vi "Generate Report.vi"(11 "Data In":T1={"Impulse Positions"=[], "No. Imp"=0, "Parameter Time Series"=[], "Parameter Impuls Series"=[], "Experiment Parameters"={"Freq"=0.0, "Vel"=0, "Acc"=0, "Stimulus"=""}, "Autosort File"=refnum, "Data File"={"Data Channels"=[], "Sample Rate"=0, "Channel List"=[]}, "Experiment data path"=path "/Macintosh HD/Users/patrick/Studium/Diploma Thesis/Data Analysis", "Image data path"=path "/Macintosh HD/Users/patrick/Studium/Diploma Thesis/Data Analysis", "LVS data path"=path "/Macintosh HD/Users/patrick/Studium/Diploma Thesis/Data Analysis", "Raw copy path"=path "/Macintosh HD/Users/patrick/Studium/Diploma Thesis/Data Analysis", "filename"="No file selected", "desaccading parameters"={"Tolerance"=0, "Acc Range"=0.0, "Sample Rate"=0, "Impulse Plane 2"=enum."Other", "Impulse dir"=FALSE}, "Experiment Parameters 2"={"Subject"="", "Strain"="", "Rotation plane"="", "Experimenter"="", "Trial"=0.0, "Time"=0.0}, "Excel"={"Excel._Application"=refnum, "Use Excel"=FALSE, "Worksheet SINE"=refnum, "Row SINE"=0, "Worksheet TRANS"=refnum, "Row TRANS"=0}, "Session Config File"=refnum, "Autosort Parameter Set"=1, "EMA Version"="", "desacc "={"Threshold 1 [Acc]"=7000.0, "Threshold 2 [% of TH1]"=60, "tolerance"=3, "Search WD "=0.1, " always use TH2"=FALSE, "Range"=2.0, "Max time"=120.0, "Min time"=20.0, "Velocity Threshold"=150}, "Cycle Nr for Saccades"={"POS"=0, "NEG"=0}, "calibration name"="No file selected", "Excel"=refnum} {"Parameter Time Series"."time offset" format="%.3f"; "Parameter Time Series"."Gain" format="%.1f"; "Parameter Time Series"."Offset" format="%.1f"; "Parameter Time Series"."List 1" items=["Motor-Pos", "Motor-Vel", "Lx Position-in-Head", "Ly Position-in-Head", "Lz Position-in-Head", "Lx Velocity-in-Head", "Ly Velocity-in-Head", "Lz Velocity-in-Head", "Ll Velocity-in-Head", "Lr Velocity-in-Head", "Lx Accel-in-Head", "Ly Accel-in-Head", "Lz Accel-in-Head", "Rx Position-in-Head", "Ry Position-in-Head", "Rz Position-in-Head", "Rx Velocity-in-Head", "Ry Velocity-in-Head", "Rz Velocity-in-Head", "Rl Velocity-in-Head", "Rr Velocity-in-Head", "Rx Accel-in-Head", "Ry Accel-in-Head", "Rz Accel-in-Head", "Global Trigger", "", "", ""]; "Parameter Impuls Series"."Gain" format="%.1f"; "Parameter Impuls Series"."Offset" format="%.1f"}) -> (3 "Data Out":T1={"Impulse Positions"=[], "No. Imp"=0, "Parameter Time Series"=[], "Parameter Impuls Series"=[], "Experiment Parameters"={"Freq"=0.0, "Vel"=0, "Acc"=0, "Stimulus"=""}, "Autosort File"=refnum, "Data File"={"Data Channels"=[], "Sample Rate"=0, "Channel List"=[]}, "Experiment data path"=path "/Macintosh HD/Users/patrick/Studium/Diploma Thesis/Data Analysis", "Image data path"=path "/Macintosh HD/Users/patrick/Studium/Diploma Thesis/Data Analysis", "LVS data path"=path "/Macintosh HD/Users/patrick/Studium/Diploma Thesis/Data Analysis", "Raw copy path"=path "/Macintosh HD/Users/patrick/Studium/Diploma Thesis/Data Analysis", "filename"="No file selected", "desaccading parameters"={"Tolerance"=0, "Acc Range"=0.0, "Sample Rate"=0, "Impulse Plane 2"=enum."Other", "Impulse dir"=FALSE}, "Experiment Parameters 2"={"Subject"="", "Strain"="", "Rotation plane"="", "Experimenter"="", "Trial"=0.0, "Time"=0.0}, "Excel"={"Excel._Application"=refnum, "Use Excel"=FALSE, "Worksheet SINE"=refnum, "Row SINE"=0, "Worksheet TRANS"=refnum, "Row TRANS"=0}, "Session Config File"=refnum, "Autosort Parameter Set"=1, "EMA Version"="", "desacc "={"Threshold 1 [Acc]"=7000.0, "Threshold 2 [% of TH1]"=60, "tolerance"=3, "Search WD "=0.1, " always use TH2"=FALSE, "Range"=2.0, "Max time"=120.0, "Min time"=20.0, "Velocity Threshold"=150}, "Cycle Nr for Saccades"={"POS"=0, "NEG"=0}, "calibration name"="No file selected", "Excel"=refnum} {"Parameter Time Series"."time offset" format="%.3f"; "Parameter Time Series"."Gain" format="%.1f"; "Parameter Time Series"."Offset" format="%.1f"; "Parameter Time Series"."List 1" items=["Motor-Pos", "Motor-Vel", "Lx Position-in-Head", "Ly Position-in-Head", "Lz Position-in-Head", "Lx Velocity-in-Head", "Ly Velocity-in-Head", "Lz Velocity-in-Head", "Ll Velocity-in-Head", "Lr Velocity-in-Head", "Lx Accel-in-Head", "Ly Accel-in-Head", "Lz Accel-in-Head", "Rx Position-in-Head", "Ry Position-in-Head", "Rz Position-in-Head", "Rx Velocity-in-Head", "Ry Velocity-in-Head", "Rz Velocity-in-Head", "Rl Velocity-in-Head", "Rr Velocity-in-Head", "Rx Accel-in-Head", "Ry Accel-in-Head", "Rz Accel-in-Head", "Global Trigger", "", "", ""]; "Parameter Impuls Series"."Gain" format="%.1f"; "Parameter Impuls Series"."Offset" format="%.1f"})   [LabVIEW 2016, in "generate report.lvlib"]
uses:
  generate report.lvlib
  core/type-defs/TD_Statemachine-Data.ctl
  <userlib>/Import Export/Excel/Excel.lvclass
  core/type-defs/TD_Time Series.ctl
  core/type-defs/TD_Impulse Parameter.ctl
  Enum_Statistical Methods Within Impulses.ctl
  Enum_Statistical Methods Across Impulses.ctl
  Enum_Report State.ctl
  <vilib>/Utility/miscctls.llb/LVRectTypeDef.ctl
  <vilib>/Utility/NIReport.llb/Append Image to Report (path wrap).vi
  <vilib>/Utility/NIReport.llb/Append Report Text (str wrap).vi
  <vilib>/Utility/NIReport.llb/NI_report.lvclass
  comm/impulse/impulse functions.lvlib
  <vilib>/Utility/NIReport.llb/NI_ReportGenerationCore.lvlib
  core/core.lvlib
panel:
  in  "5 PeakVel SD":dbl format="%#_13g"
  in  "5 PeakVel":dbl format="%#_13g"
  in  "4 PeakVel SD":dbl format="%#_13g"
  in  "4 PeakVel":dbl format="%#_13g"
  in  "2 PeakVel":dbl format="%#_13g"
  in  "2 PeakVel SD":dbl format="%#_13g"
  in  "3 PeakVel":dbl format="%#_13g"
  in  "3 PeakVel SD":dbl format="%#_13g"
  in  "1 PeakVel":dbl format="%#_13g"
  in  "1 PeakVel SD":dbl format="%#_13g"
  in  "0 PeakVel SD":dbl format="%#_13g"
  in  "0 PeakVel":dbl format="%#_13g"
  out "5 N":i32
  out "4 N":i32
  out "3 N":i32
  out "2 N":i32
  out "1 N":i32
  out "0 N":i32
  out "Stimulus":string
  out "3 SD":dbl=-0.0 format="%.2f"
  out "2 SD":dbl=-0.0 format="%.2f"
  out "0 SD":dbl=-0.0 format="%.2f"
  out "1 SD":dbl=-0.0 format="%.2f"
  out "4 SD":dbl=-0.0 format="%.2f"
  out "5 SD":dbl=-0.0 format="%.2f"
  out "3 Gain":dbl=nan format="%.2f"
  out "2 Gain":dbl=nan format="%.2f"
  out "0 Gain":dbl=nan format="%.2f"
  out "1 Gain":dbl=nan format="%.2f"
  in  "Patient ID":string
  out "4 Gain":dbl=nan format="%.2f"
  out "5 Gain":dbl=nan format="%.2f"
  out "5":cluster{dbl, dbl, "Impulses":dbl[][]}(graph)={0.0, 2.5, "Impulses"=[]}
  out "3":cluster{dbl, dbl, "Impulses":dbl[][]}(graph)={0.0, 2.5, "Impulses"=[]}
  out "4":cluster{dbl, dbl, "Impulses":dbl[][]}(graph)={0.0, 2.5, "Impulses"=[]}
  out "2":cluster{dbl, dbl, "Impulses":dbl[][]}(graph)={0.0, 2.5, "Impulses"=[]}
  out "1":cluster{dbl, dbl, "Impulses":dbl[][]}(graph)={0.0, 2.5, "Impulses"=[]}
  out "0":cluster{dbl, dbl, "Impulses":dbl[][]}(graph)={0.0, 2.5, "Impulses"=[]}
  in  "Save to Excel (legacy)":bool
  in  "PS - RollPitch":bool
  in  "PS - EyHy":bool
  in  "PS - EyHlr":bool
  in  "PS - All3D":bool
  out "Analysis Required?":bool
  in  "Impulse Group Gain Method":T4
  in  "Impulse Gain Method":T5=enum."Median"
  in  "Save to Excel":bool
  in  "Printer Select":string(combo) caption="Selected Printer"
  in  "print horizontal":bool
  in  "Save to File":bool
  in  "print all":bool
  in  "Graph Properties":T6(array[cluster])=[{"Plot Traces"=[{"Color Box"=6618880, "Boolean"=TRUE, "List 2"=1, "Boolean 2"=FALSE, "Boolean 3"=FALSE, "Offset"=0.0, "Gain"=1.0}, {"Color Box"=4467455, "Boolean"=TRUE, "List 2"=13, "Boolean 2"=TRUE, "Boolean 3"=FALSE, "Offset"=0.0, "Gain"=1.0}, {"Color Box"=16711680, "Boolean"=TRUE, "List 2"=21, "Boolean 2"=TRUE, "Boolean 3"=FALSE, "Offset"=0.0, "Gain"=1.0}], "Gain Calculations"={"Threshold Trace"=1, "Min Thresh/%"=0.2, "Max Thresh/%"=0.8, "Gain calculated by dividing"=13, "Gain Range"=enum."Best Est", "Pre-peak-ms"=30.0, "by"=1}, "Impulse Plane"=enum."Yaw", "Impulse Direction"=TRUE}, {"Plot Traces"=[{"Color Box"=6618880, "Boolean"=TRUE, "List 2"=1, "Boolean 2"=TRUE, "Boolean 3"=FALSE, "Offset"=0.0, "Gain"=1.0}, {"Color Box"=1966335, "Boolean"=TRUE, "List 2"=13, "Boolean 2"=FALSE, "Boolean 3"=FALSE, "Offset"=0.0, "Gain"=1.0}, {"Color Box"=16711680, "Boolean"=TRUE, "List 2"=21, "Boolean 2"=FALSE, "Boolean 3"=FALSE, "Offset"=0.0, "Gain"=1.0}], "Gain Calculations"={"Threshold Trace"=1, "Min Thresh/%"=0.2, "Max Thresh/%"=0.8, "Gain calculated by dividing"=13, "Gain Range"=enum."Best Est", "Pre-peak-ms"=30.0, "by"=1}, "Impulse Plane"=enum."Yaw", "Impulse Direction"=FALSE}, {"Plot Traces"=[{"Color Box"=4652800, "Boolean"=TRUE, "List 2"=6, "Boolean 2"=TRUE, "Boolean 3"=FALSE, "Offset"=0.0, "Gain"=1.0}, {"Color Box"=1966335, "Boolean"=TRUE, "List 2"=14, "Boolean 2"=FALSE, "Boolean 3"=FALSE, "Offset"=0.0, "Gain"=1.0}, {"Color Box"=16722474, "Boolean"=TRUE, "List 2"=22, "Boolean 2"=FALSE, "Boolean 3"=FALSE, "Offset"=0.0, "Gain"=1.0}], "Gain Calculations"={"Threshold Trace"=6, "Min Thresh/%"=0.2, "Max Thresh/%"=0.8, "Gain calculated by dividing"=14, "Gain Range"=enum."Best Est", "Pre-peak-ms"=30.0, "by"=6}, "Impulse Plane"=enum."LARP", "Impulse Direction"=FALSE}, {"Plot Traces"=[{"Color Box"=4652800, "Boolean"=TRUE, "List 2"=7, "Boolean 2"=FALSE, "Boolean 3"=FALSE, "Offset"=0.0, "Gain"=1.0}, {"Color Box"=1966335, "Boolean"=TRUE, "List 2"=15, "Boolean 2"=TRUE, "Boolean 3"=FALSE, "Offset"=0.0, "Gain"=1.0}, {"Color Box"=16722474, "Boolean"=TRUE, "List 2"=23, "Boolean 2"=TRUE, "Boolean 3"=FALSE, "Offset"=0.0, "Gain"=1.0}], "Gain Calculations"={"Threshold Trace"=7, "Min Thresh/%"=0.2, "Max Thresh/%"=0.8, "Gain calculated by dividing"=15, "Gain Range"=enum."Best Est", "Pre-peak-ms"=30.0, "by"=7}, "Impulse Plane"=enum."RALP", "Impulse Direction"=TRUE}, {"Plot Traces"=[{"Color Box"=4652800, "Boolean"=TRUE, "List 2"=7, "Boolean 2"=TRUE, "Boolean 3"=FALSE, "Offset"=0.0, "Gain"=1.0}, {"Color Box"=1966335, "Boolean"=TRUE, "List 2"=15, "Boolean 2"=FALSE, "Boolean 3"=FALSE, "Offset"=0.0, "Gain"=1.0}, {"Color Box"=16722474, "Boolean"=TRUE, "List 2"=23, "Boolean 2"=FALSE, "Boolean 3"=FALSE, "Offset"=0.0, "Gain"=1.0}], "Gain Calculations"={"Threshold Trace"=7, "Min Thresh/%"=0.2, "Max Thresh/%"=0.8, "Gain calculated by dividing"=15, "Gain Range"=enum."Best Est", "Pre-peak-ms"=30.0, "by"=7}, "Impulse Plane"=enum."RALP", "Impulse Direction"=FALSE}, {"Plot Traces"=[{"Color Box"=4652800, "Boolean"=TRUE, "List 2"=6, "Boolean 2"=FALSE, "Boolean 3"=FALSE, "Offset"=0.0, "Gain"=1.0}, {"Color Box"=1966335, "Boolean"=TRUE, "List 2"=14, "Boolean 2"=TRUE, "Boolean 3"=FALSE, "Offset"=0.0, "Gain"=1.0}, {"Color Box"=16722474, "Boolean"=TRUE, "List 2"=22, "Boolean 2"=TRUE, "Boolean 3"=FALSE, "Offset"=0.0, "Gain"=1.0}], "Gain Calculations"={"Threshold Trace"=6, "Min Thresh/%"=0.2, "Max Thresh/%"=0.8, "Gain calculated by dividing"=14, "Gain Range"=enum."Best Est", "Pre-peak-ms"=30.0, "by"=6}, "Impulse Plane"=enum."LARP", "Impulse Direction"=TRUE}] {"Gain Calculations"."by" items=["-", "Hz Velocity-in-Head", "-", "Hy Velocity-in-Head", "-", "Hx Velocity-in-Head", "Hl Velocity-in-Head", "Hr Velocity-in-Head", "-", "Ly Position-in-Head", "Lz Position-in-Head", "-", "Ly Velocity-in-Head", "Lz Velocity-in-Head", "-", "Hx Acceleration-in-Head", "Hy Acceleration-in-Head", "Hz Acceleration-in-Head", "Hl Acceleration-in-Head", "Hr Acceleration-in-Head", "-", "Ly Acceleration-in-Head", "Lz Acceleration-in-Head", "-"]; "Gain Calculations"."Pre-peak-ms" format="%.2f"; "Gain Calculations"."Gain calculated by dividing" items=["-", "Hz Velocity-in-Head", "-", "Hy Velocity-in-Head", "-", "Hx Velocity-in-Head", "Hl Velocity-in-Head", "Hr Velocity-in-Head", "-", "Ly Position-in-Head", "Lz Position-in-Head", "-", "Ly Velocity-in-Head", "Lz Velocity-in-Head", "-", "Hx Acceleration-in-Head", "Hy Acceleration-in-Head", "Hz Acceleration-in-Head", "Hl Acceleration-in-Head", "Hr Acceleration-in-Head", "-", "Ly Acceleration-in-Head", "Lz Acceleration-in-Head", "-"]; "Gain Calculations"."Max Thresh/%" format="%.2f"; "Gain Calculations"."Min Thresh/%" format="%.2f"; "Gain Calculations"."Threshold Trace" items=["-", "Hz Velocity-in-Head", "-", "Hy Velocity-in-Head", "-", "Hx Velocity-in-Head", "Hl Velocity-in-Head", "Hr Velocity-in-Head", "-", "Ly Position-in-Head", "Lz Position-in-Head", "-", "Ly Velocity-in-Head", "Lz Velocity-in-Head", "-", "Hx Acceleration-in-Head", "Hy Acceleration-in-Head", "Hz Acceleration-in-Head", "Hl Acceleration-in-Head", "Hr Acceleration-in-Head", "-", "Ly Acceleration-in-Head", "Lz Acceleration-in-Head", "-"]; "Plot Traces"."Gain" format="%.1f"; "Plot Traces"."Offset" format="%.1f"; "Plot Traces"."List 2" items=["-", "Hz Velocity-in-Head", "-", "Hy Velocity-in-Head", "-", "Hx Velocity-in-Head", "Hl Velocity-in-Head", "Hr Velocity-in-Head", "-", "Ly Position-in-Head", "Lz Position-in-Head", "-", "Ly Velocity-in-Head", "Lz Velocity-in-Head", "-", "Hx Acceleration-in-Head", "Hy Acceleration-in-Head", "Hz Acceleration-in-Head", "Hl Acceleration-in-Head", "Hr Acceleration-in-Head", "-", "Ly Acceleration-in-Head", "Lz Acceleration-in-Head", "-"]}
  # "Canal Plane Responses"
  # "RIGHT"
  # "LEFT"
  # "Horizontal"
  # "Horizontal"
  # "Anterior"
  # "Anterior"
  # "Posterior"
  # "Posterior"
  # "Gain Calculation Presets"
  # "Copyright Americo A. Migliaccio (c) 2002 All Rights Reserved by Author"
  # "Gain Methods for 'Best Est' Calculation"
  # "-"
  # "+"
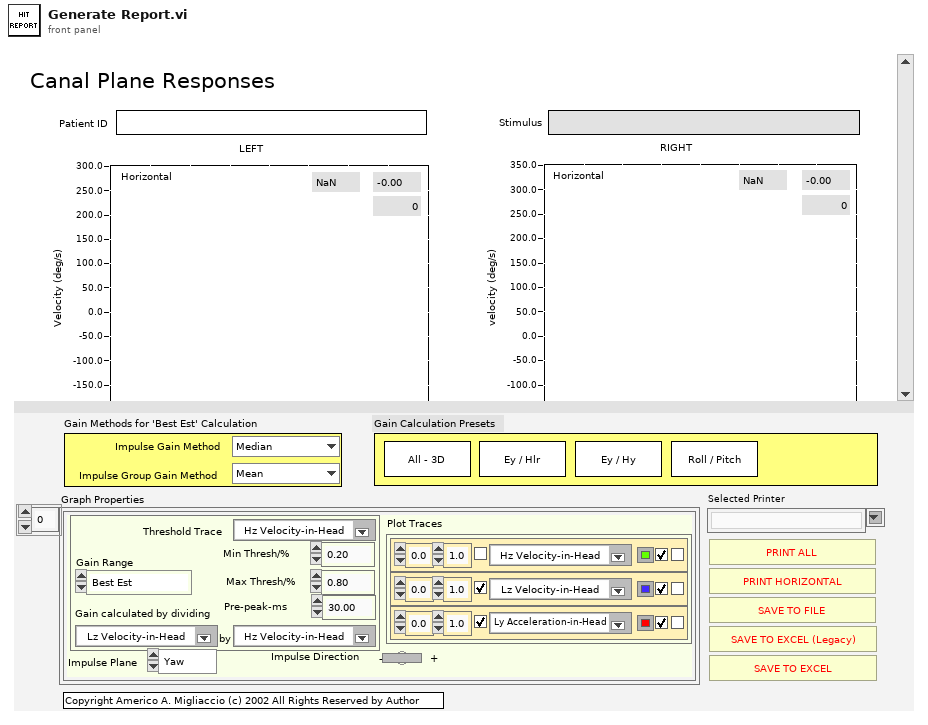
[diagram p1: front panel]
types:
  T1 = typedef "core.lvlib/TD_Statemachine-Data.ctl" = cluster{"Impulse Positions":cluster{"Start":i32, "End":i32, "Impulse Plane":enum16{"Other", "Yaw", "Pitch", "Roll", "LARP", "RALP"}, "Impulse Direction +ve?":bool, "Time offset":i32, "Amplitude offset":dbl}[], "No. Imp":i32, "Parameter Time Series":T2, "Parameter Impuls Series":T3, "Experiment Parameters":cluster{"Freq":dbl, "Vel":i32, "Acc":i32, "Stimulus":string}, "Autosort File":refnum<file>, "Data File":cluster{"Data Channels":dbl[][], "Sample Rate":i32, "Channel List":string[]}, "Experiment data path":path, "Image data path":path, "LVS data path":path, "Raw copy path":path, "filename":string, "desaccading parameters":cluster{"Tolerance":i32, "Acc Range":dbl, "Sample Rate":i32, "Impulse Plane 2":enum16{"Other", "Yaw", "Pitch", "Roll", "LARP", "RALP"}, "Impulse dir":bool}, "Experiment Parameters 2":cluster{"Subject":string, "Strain":string, "Rotation plane":string, "Experimenter":string, "Trial":dbl, "Time":dbl}, "Excel":cluster{"Excel._Application":refnum<k7>, "Use Excel":bool, "Worksheet SINE":refnum<k7>, "Row SINE":i32, "Worksheet TRANS":refnum<k7>, "Row TRANS":i32}, "Session Config File":refnum<file>, "Autosort Parameter Set":i32, "EMA Version":string, "desacc ":cluster{"Threshold 1 [Acc]":dbl, "Threshold 2 [% of TH1]":i32, "tolerance":i32, "Search WD ":dbl, " always use TH2":bool, "Range":dbl, "Max time":dbl, "Min time":dbl, "Velocity Threshold":i32}, "Cycle Nr for Saccades":cluster{"POS":i32, "NEG":i32}, "calibration name":string, "Excel":refnum<class "Excel.lvclass">}
  T2 = typedef "core.lvlib/TD_Time Series.ctl" = cluster{"time offset":dbl, "Offset":dbl, "Gain":dbl, "inverse":bool, "filter data":bool, "dots":bool, "interpolate":bool, "List 1":u16, "Color Box":u32, "Boolean":bool}[]
  T3 = typedef "core.lvlib/TD_Impulse Parameter.ctl" = cluster{"Color":u32, "Visible":bool, "Channel":u16, "Invert":bool, "Desaccade":bool, "Offset":dbl, "Gain":dbl}[]
  T4 = typedef "generate report.lvlib/Enum_Statistical Methods Across Impulses.ctl" = enum16{"Mean", "Median"}
  T5 = typedef "generate report.lvlib/Enum_Statistical Methods Within Impulses.ctl" = enum16{"Max", "Mean", "Median"}
  T6 = cluster{"Plot Traces":cluster{"Color Box":u32, "Boolean":bool, "List 2":u16, "Boolean 2":bool, "Boolean 3":bool, "Offset":dbl, "Gain":dbl}[], "Gain Calculations":cluster{"Threshold Trace":u16, "Min Thresh/%":dbl, "Max Thresh/%":dbl, "Gain calculated by dividing":u16, "Gain Range":enum16{"Peak %", "Best Est", "Thresh"}, "Pre-peak-ms":dbl, "by":u16}, "Impulse Plane":enum16{"Other", "Yaw", "Pitch", "Roll", "LARP", "RALP"}, "Impulse Direction":bool}[]
  T7 = typedef "generate report.lvlib/Enum_Report State.ctl" = enum16{"Idle", "Initialize", "Quit", "Analyze", "Print All", "Print Horizontal", "Save Text File", "Save To Excel", "Save To Excel (legacy)"}
  T8 = enum16{"Standard Report", "HTML", "Word", "Excel"}
  T9 = cluster{"left":i16, "top":i16, "right":i16, "bottom":i16}
  T10 = typedef "LVRectTypeDef.ctl" = cluster{"Left":i16, "Top":i16, "Right":i16, "Bottom":i16}
  T11 = enum16{"open", "replace", "create", "open or create", "replace or create", "replace or create with confirmation"}
  T12 = cluster{"Threshold 1 [Acc]":dbl, "Threshold 2 [% of TH1]":i32, "tolerance":i32, "Search WD ":dbl, " always use TH2":bool, "Range":dbl, "Max time":dbl, "Min time":dbl, "Velocity Threshold":i32}
  T13 = cluster{"Data Channels":dbl[][], "Sample Rate":i32, "Channel List":string[]}
  T14 = cluster{"Start":i32, "End":i32, "Impulse Plane":enum16{"Other", "Yaw", "Pitch", "Roll", "LARP", "RALP"}, "Impulse Direction +ve?":bool, "Time offset":i32, "Amplitude offset":dbl}[]
  T15 = cluster{"Impulse Gain Method":T5, "Impulse Group Gain Method":T4}
  T16 = enum16{"Other", "Yaw", "Pitch", "Roll", "LARP", "RALP"}
  T17 = cluster{"Color Box":u32, "Boolean":bool, "List 2":u16, "Boolean 2":bool, "Boolean 3":bool, "Offset":dbl, "Gain":dbl}[]
  T18 = typedef "imagedata.ctl" = cluster{"image type":i32, "image depth":i32, "image":u8[], "mask":u8[], "colors":u32[], "Rectangle":cluster{"left":i16, "top":i16, "right":i16, "bottom":i16}}
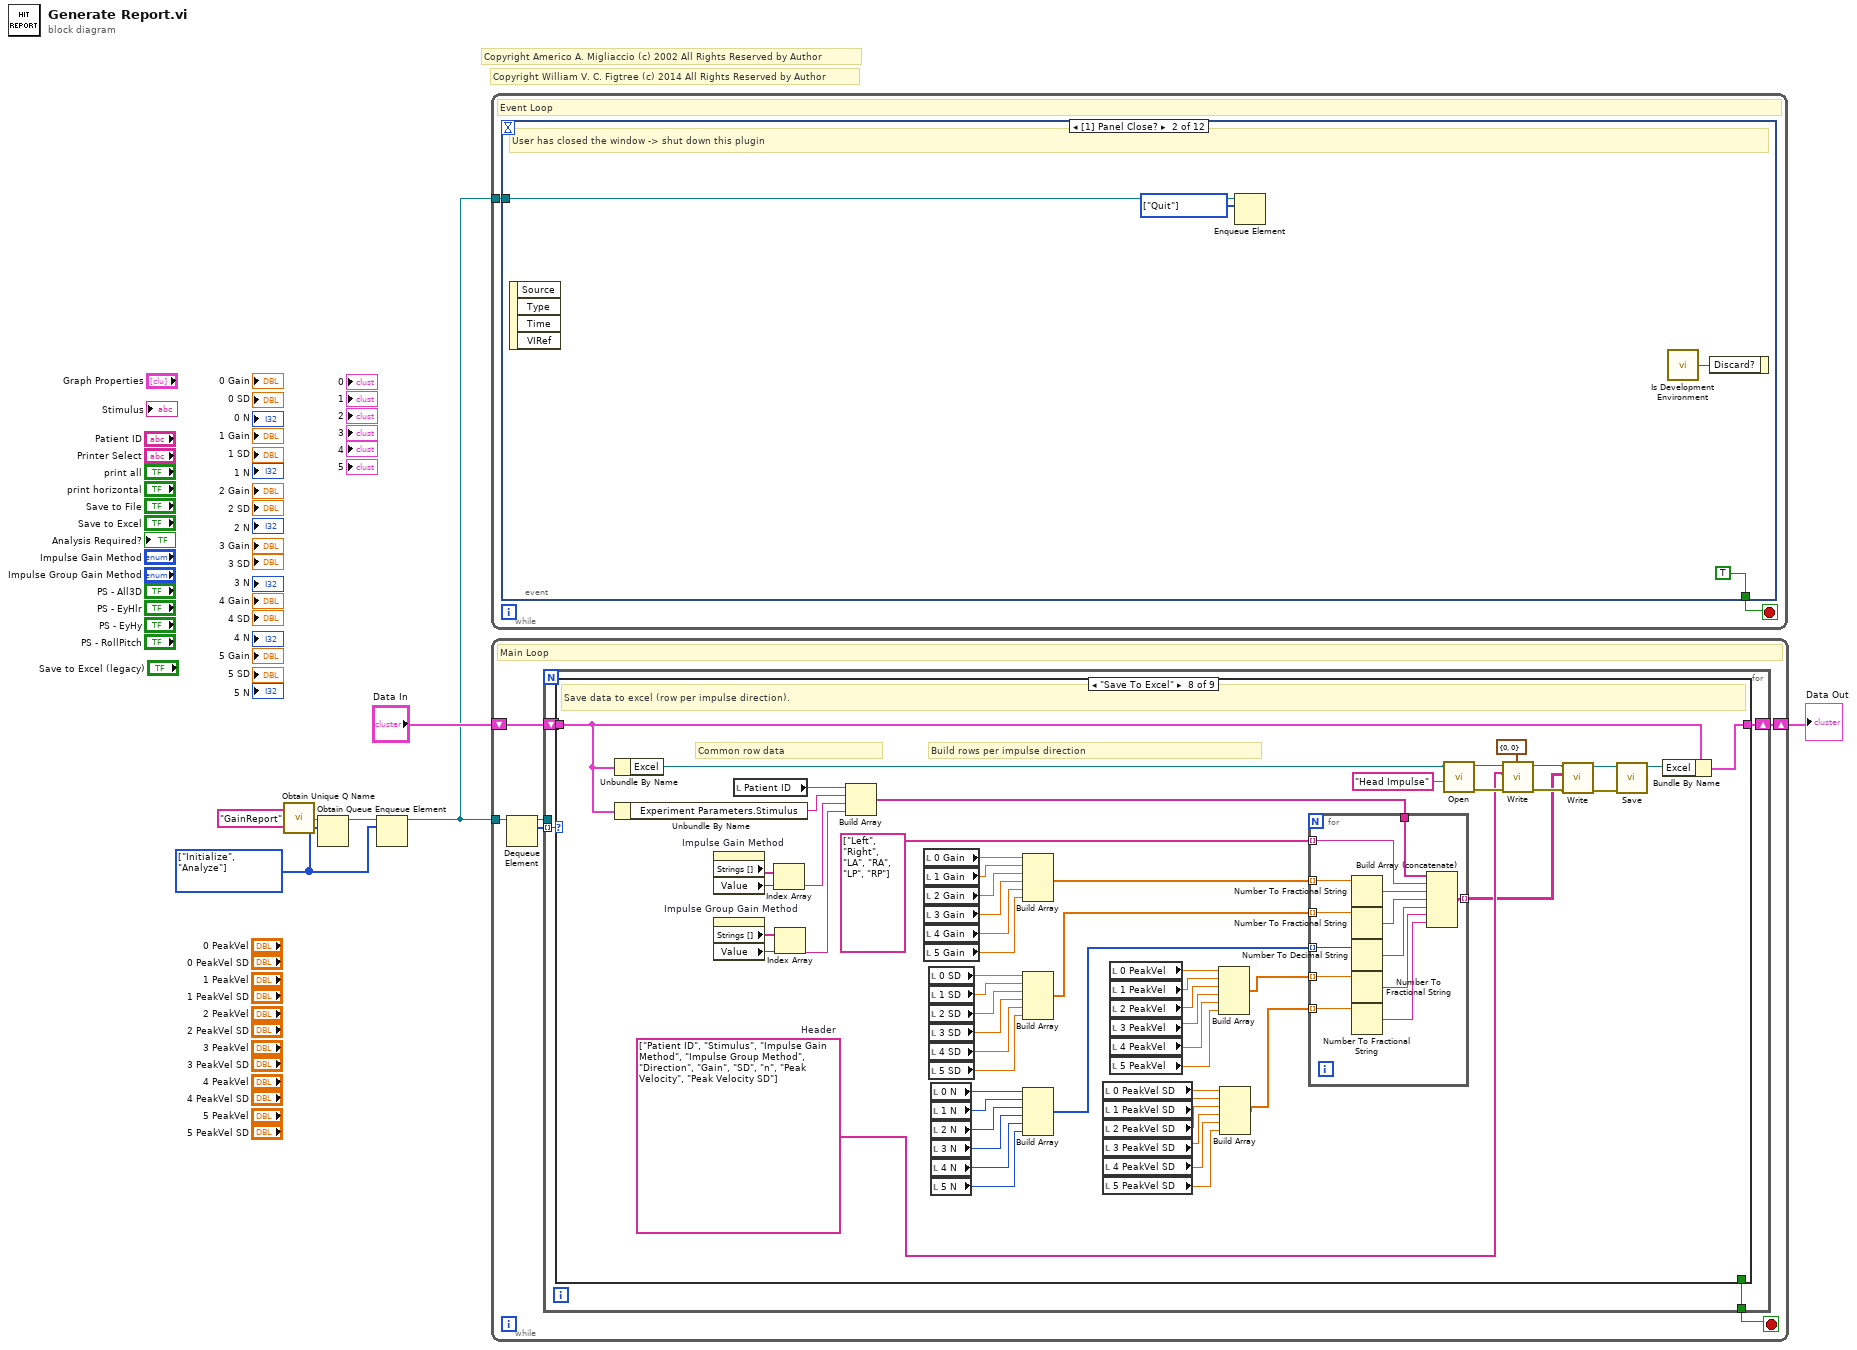
[diagram p0: block diagram]
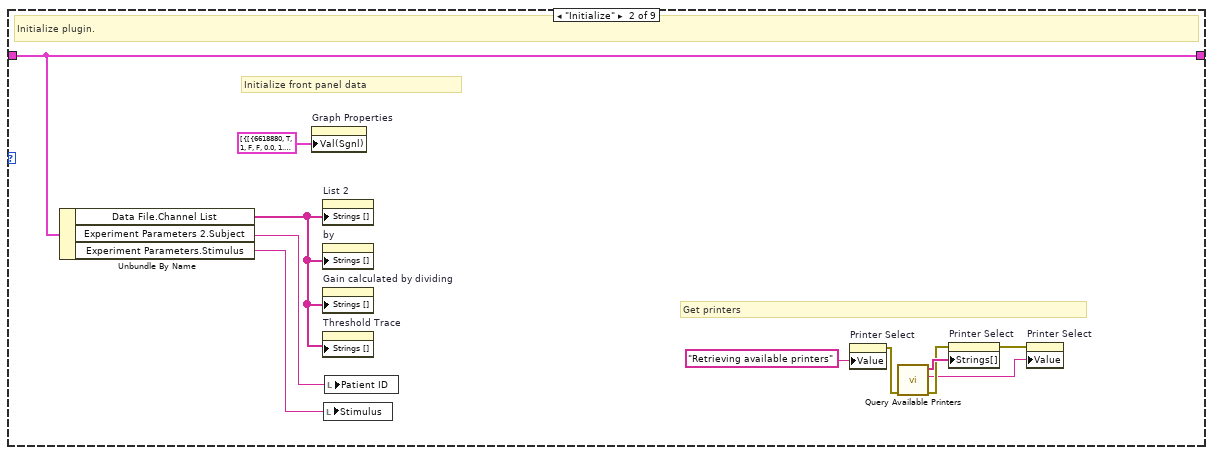
[diagram p3: hidden frame]
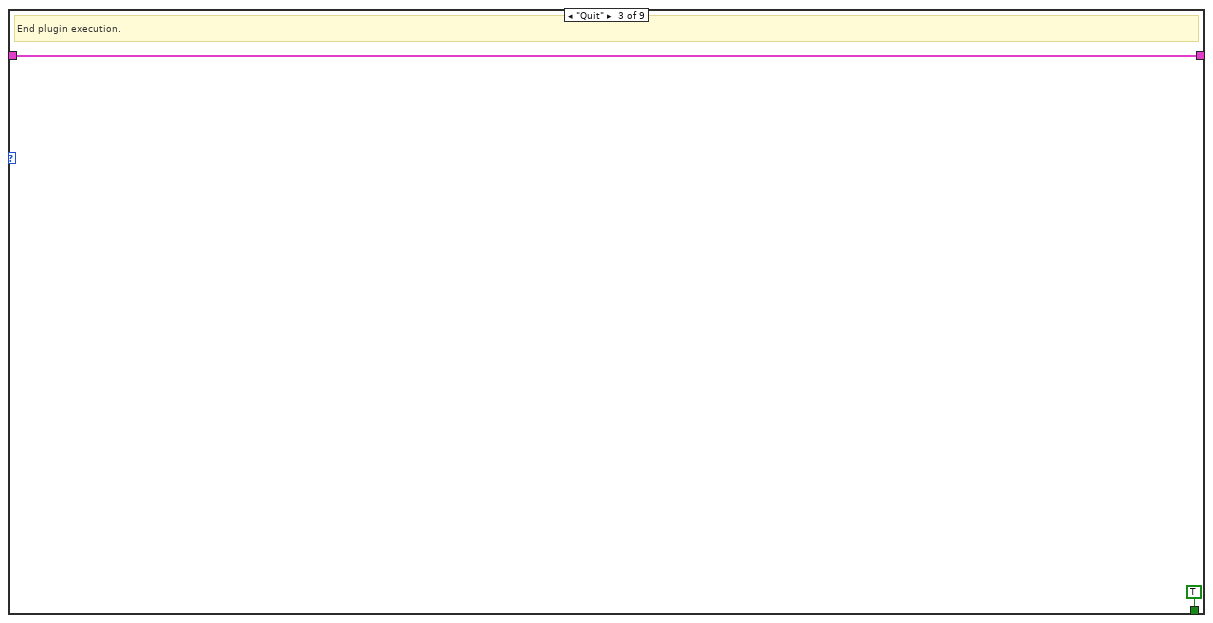
[diagram p4: hidden frame]
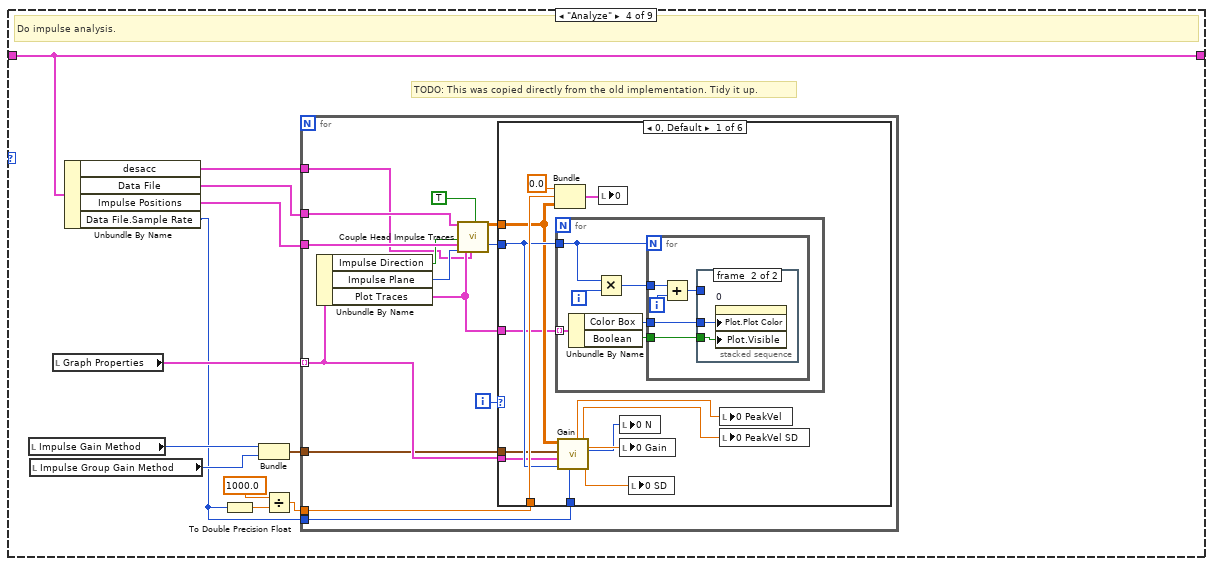
[diagram p5: hidden frame]
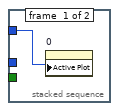
[diagram p6: hidden frame]
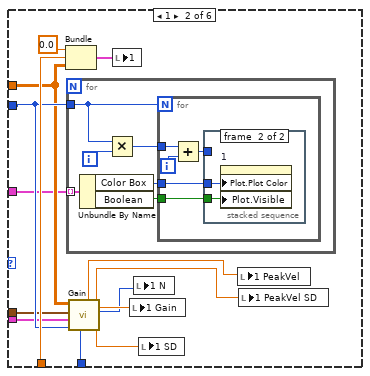
[diagram p7: hidden frame]
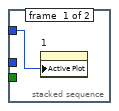
[diagram p8: hidden frame]
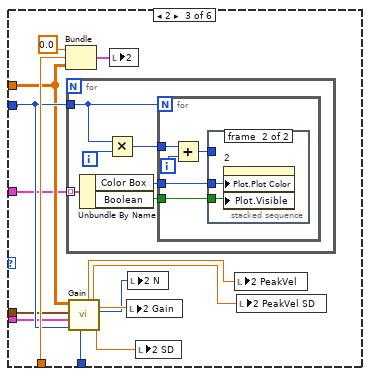
[diagram p9: hidden frame]
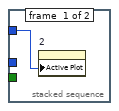
[diagram p10: hidden frame]
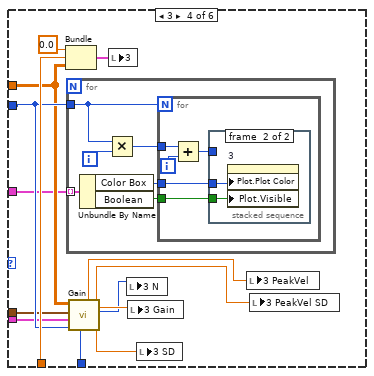
[diagram p11: hidden frame]
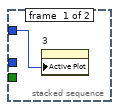
[diagram p12: hidden frame]
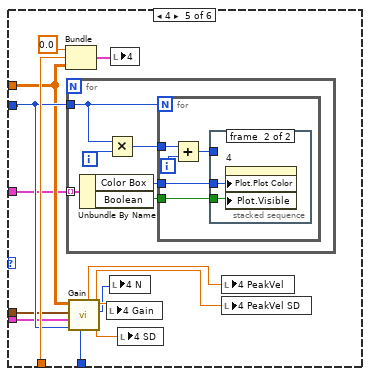
[diagram p13: hidden frame]
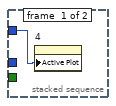
[diagram p14: hidden frame]
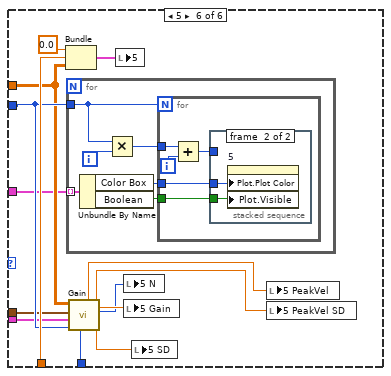
[diagram p15: hidden frame]
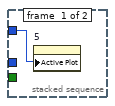
[diagram p16: hidden frame]
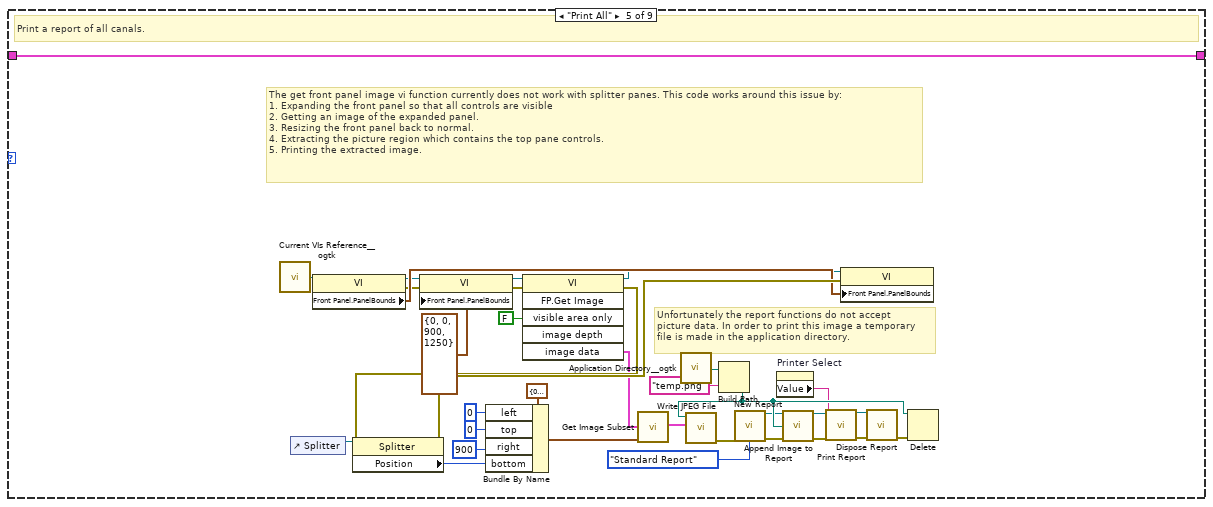
[diagram p17: hidden frame]
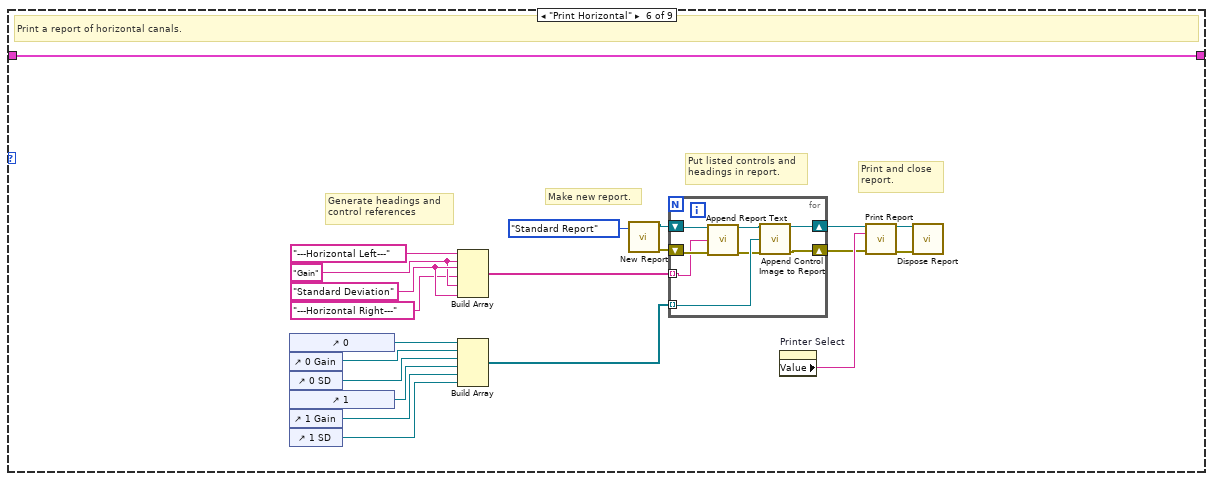
[diagram p18: hidden frame]
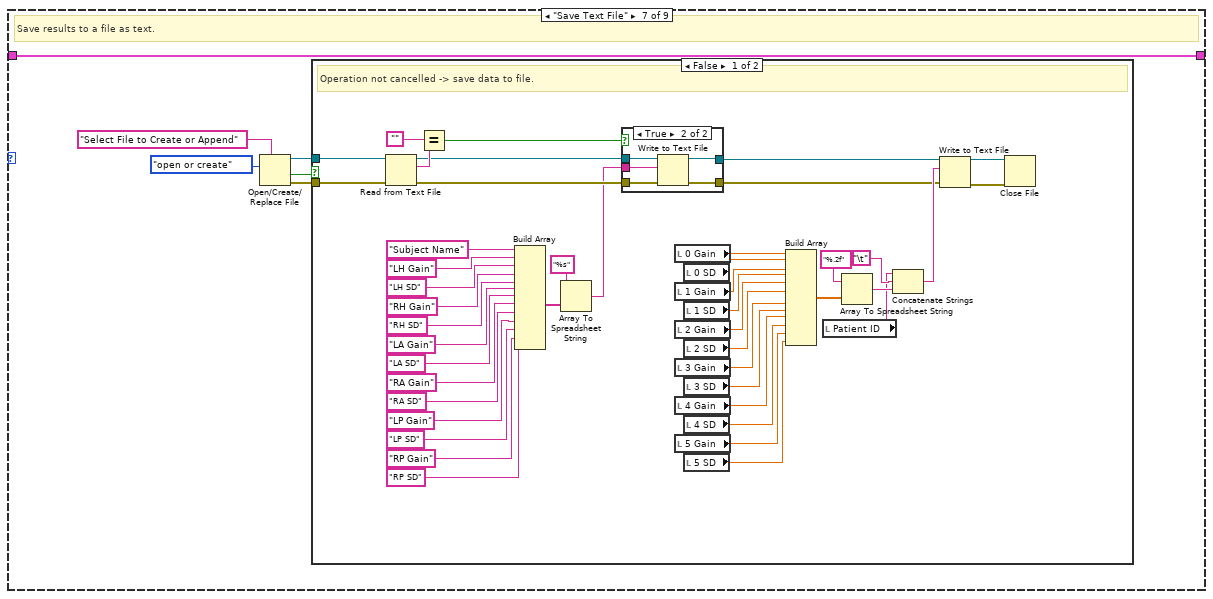
[diagram p19: hidden frame]
diagram:
  w4 = T7[] [enum."Initialize", enum."Analyze"] items=["Idle", "Initialize", "Quit", "Analyze", "Print All", "Print Horizontal", "Save Text File", "Save To Excel", "Save To Excel (legacy)"] ("Array")
  # "Copyright William V. C. Figtree (c) 2014 All Rights Reserved by Author"
  # "Copyright Americo A. Migliaccio (c) 2002 All Rights Reserved by Author"
  n1 = call <userlib>:"Obtain Unique Q Name.vi"("Queue"="GainReport") -> ("Q Name"=w7:string)  [unwired: 4 in]
  n2 = Obtain Queue(name (unnamed)=w7, element data type=w4) -> (queue out=w5:refnum<queue>)  [unwired: 3 in, 2 out]
  n3 = Enqueue Element(queue=w5, element=w4) -> (queue out=w2:refnum<queue>)  [unwired: 2 in, 2 out]
  n4 = while {
    tunnel: w2 -> [w8]
    stop <- w9 stop-if-true
    # "Event Loop"
    n5 = event shown="[1] Panel Close?" {
      selector: _ -> [_ _ _ _ _ _ _ _ _ _ _ _]
      dyn-events: _ -> [_ _ _ _ _ _ _ _ _ _ _ _]
      timeout: _ -> [_ _ _ _ _ _ _ _ _ _ _ _]
      tunnel: [_ TRUE _ _ _ _ _ _ _ _ _ _] -> w9
      tunnel: w8 -> [_ w11 w15 _ _ _ _ w21 w23 w25 w27 w29]
      event Timeout {
        n6 = event-data() -> ()  [unwired: 1 in, 3 out]
      }
      event Panel Close? {
        w10 = T7[] [enum."Quit"] items=["Idle", "Initialize", "Quit", "Analyze", "Print All", "Print Horizontal", "Save Text File", "Save To Excel", "Save To Excel (legacy)"] ("element")
        # "User has closed the window -> shut down this plugin"
        n7 = event-data() -> ()  [unwired: 1 in, 4 out]
        n8 = Enqueue Element(queue=w11, element=w10) -> ()  [unwired: 2 in, 3 out]
        n9 = call <userlib>:"Is Development Environment.vi"() -> ("exe?"=w12:bool)  [unwired: 5 in]
        n10 = event-data("Discard?"=w12) -> ()  [unwired: 1 in, 1 out]
      }
      event "Graph Properties": Value Change {
        w14 = T7[] [enum."Analyze"] items=["Idle", "Initialize", "Quit", "Analyze", "Print All", "Print Horizontal", "Save Text File", "Save To Excel", "Save To Excel (legacy)"] ("element")
        # "front panel edits -> prompt anaysis refresh"
        n11 = event-data() -> ()  [unwired: 1 in, 6 out]
        n12 = Enqueue Element(queue=w15, element=w14) -> ()  [unwired: 2 in, 3 out]
      }
      event "PS - All3D": Value Change {
        # "Apply selected preset graph properties"
        n13 = event-data() -> ()  [unwired: 1 in, 6 out]
        n14 = property on="Graph Properties" class="Arr (strict)"("Val(Sgnl)"=T6 [{"Plot Traces"=[{"Color Box"=6618880, "Boolean"=TRUE, "List 2"=1, "Boolean 2"=FALSE, "Boolean 3"=FALSE, "Offset"=0.0, "Gain"=1.0}, {"Color Box"=4467455, "Boolean"=TRUE, "List 2"=13, "Boolean 2"=TRUE, "Boolean 3"=FALSE, "Offset"=0.0, "Gain"=1.0}, {"Color Box"=16711680, "Boolean"=FALSE, "List 2"=21, "Boolean 2"=TRUE, "Boolean 3"=FALSE, "Offset"=0.0, "Gain"=1.0}], "Gain Calculations"={"Threshold Trace"=1, "Min Thresh/%"=0.2, "Max Thresh/%"=0.8, "Gain calculated by dividing"=13, "Gain Range"=enum."Best Est", "Pre-peak-ms"=30.0, "by"=1}, "Impulse Plane"=enum."Yaw", "Impulse Direction"=TRUE}, {"Plot Traces"=[{"Color Box"=6618880, "Boolean"=TRUE, "List 2"=1, "Boolean 2"=TRUE, "Boolean 3"=FALSE, "Offset"=0.0, "Gain"=1.0}, {"Color Box"=1966335, "Boolean"=TRUE, "List 2"=13, "Boolean 2"=FALSE, "Boolean 3"=FALSE, "Offset"=0.0, "Gain"=1.0}, {"Color Box"=16711680, "Boolean"=FALSE, "List 2"=21, "Boolean 2"=FALSE, "Boolean 3"=FALSE, "Offset"=0.0, "Gain"=1.0}], "Gain Calculations"={"Threshold Trace"=1, "Min Thresh/%"=0.2, "Max Thresh/%"=0.8, "Gain calculated by dividing"=13, "Gain Range"=enum."Best Est", "Pre-peak-ms"=30.0, "by"=1}, "Impulse Plane"=enum."Yaw", "Impulse Direction"=FALSE}, {"Plot Traces"=[{"Color Box"=4652800, "Boolean"=TRUE, "List 2"=6, "Boolean 2"=TRUE, "Boolean 3"=FALSE, "Offset"=0.0, "Gain"=1.0}, {"Color Box"=1966335, "Boolean"=TRUE, "List 2"=14, "Boolean 2"=FALSE, "Boolean 3"=FALSE, "Offset"=0.0, "Gain"=1.0}, {"Color Box"=16722474, "Boolean"=FALSE, "List 2"=22, "Boolean 2"=FALSE, "Boolean 3"=FALSE, "Offset"=0.0, "Gain"=1.0}], "Gain Calculations"={"Threshold Trace"=6, "Min Thresh/%"=0.2, "Max Thresh/%"=0.8, "Gain calculated by dividing"=14, "Gain Range"=enum."Best Est", "Pre-peak-ms"=30.0, "by"=6}, "Impulse Plane"=enum."LARP", "Impulse Direction"=FALSE}, {"Plot Traces"=[{"Color Box"=4652800, "Boolean"=TRUE, "List 2"=7, "Boolean 2"=FALSE, "Boolean 3"=FALSE, "Offset"=0.0, "Gain"=1.0}, {"Color Box"=1966335, "Boolean"=TRUE, "List 2"=15, "Boolean 2"=TRUE, "Boolean 3"=FALSE, "Offset"=0.0, "Gain"=1.0}, {"Color Box"=16722474, "Boolean"=FALSE, "List 2"=23, "Boolean 2"=TRUE, "Boolean 3"=FALSE, "Offset"=0.0, "Gain"=1.0}], "Gain Calculations"={"Threshold Trace"=7, "Min Thresh/%"=0.2, "Max Thresh/%"=0.8, "Gain calculated by dividing"=15, "Gain Range"=enum."Best Est", "Pre-peak-ms"=30.0, "by"=7}, "Impulse Plane"=enum."RALP", "Impulse Direction"=TRUE}, {"Plot Traces"=[{"Color Box"=4652800, "Boolean"=TRUE, "List 2"=7, "Boolean 2"=TRUE, "Boolean 3"=FALSE, "Offset"=0.0, "Gain"=1.0}, {"Color Box"=1966335, "Boolean"=TRUE, "List 2"=15, "Boolean 2"=FALSE, "Boolean 3"=FALSE, "Offset"=0.0, "Gain"=1.0}, {"Color Box"=16722474, "Boolean"=FALSE, "List 2"=23, "Boolean 2"=FALSE, "Boolean 3"=FALSE, "Offset"=0.0, "Gain"=1.0}], "Gain Calculations"={"Threshold Trace"=7, "Min Thresh/%"=0.2, "Max Thresh/%"=0.8, "Gain calculated by dividing"=15, "Gain Range"=enum."Best Est", "Pre-peak-ms"=30.0, "by"=7}, "Impulse Plane"=enum."RALP", "Impulse Direction"=FALSE}, {"Plot Traces"=[{"Color Box"=4652800, "Boolean"=TRUE, "List 2"=6, "Boolean 2"=FALSE, "Boolean 3"=FALSE, "Offset"=0.0, "Gain"=1.0}, {"Color Box"=1966335, "Boolean"=TRUE, "List 2"=14, "Boolean 2"=TRUE, "Boolean 3"=FALSE, "Offset"=0.0, "Gain"=1.0}, {"Color Box"=16722474, "Boolean"=FALSE, "List 2"=22, "Boolean 2"=TRUE, "Boolean 3"=FALSE, "Offset"=0.0, "Gain"=1.0}], "Gain Calculations"={"Threshold Trace"=6, "Min Thresh/%"=0.2, "Max Thresh/%"=0.8, "Gain calculated by dividing"=14, "Gain Range"=enum."Best Est", "Pre-peak-ms"=30.0, "by"=6}, "Impulse Plane"=enum."LARP", "Impulse Direction"=TRUE}] ("Graph Properties")) -> ()  [unwired: 2 in, 2 out]
      }
      event "PS - EyHlr": Value Change {
        # "Apply selected preset graph properties"
        n15 = event-data() -> ()  [unwired: 1 in, 6 out]
        n16 = property on="Graph Properties" class="Arr (strict)"("Val(Sgnl)"=T6 [{"Plot Traces"=[{"Color Box"=6618880, "Boolean"=TRUE, "List 2"=1, "Boolean 2"=FALSE, "Boolean 3"=FALSE, "Offset"=0.0, "Gain"=1.0}, {"Color Box"=4467455, "Boolean"=TRUE, "List 2"=13, "Boolean 2"=TRUE, "Boolean 3"=FALSE, "Offset"=0.0, "Gain"=1.0}, {"Color Box"=16711680, "Boolean"=FALSE, "List 2"=21, "Boolean 2"=TRUE, "Boolean 3"=FALSE, "Offset"=0.0, "Gain"=1.0}], "Gain Calculations"={"Threshold Trace"=1, "Min Thresh/%"=0.2, "Max Thresh/%"=0.8, "Gain calculated by dividing"=13, "Gain Range"=enum."Best Est", "Pre-peak-ms"=30.0, "by"=1}, "Impulse Plane"=enum."Yaw", "Impulse Direction"=TRUE}, {"Plot Traces"=[{"Color Box"=6618880, "Boolean"=TRUE, "List 2"=1, "Boolean 2"=TRUE, "Boolean 3"=FALSE, "Offset"=0.0, "Gain"=1.0}, {"Color Box"=1966335, "Boolean"=TRUE, "List 2"=13, "Boolean 2"=FALSE, "Boolean 3"=FALSE, "Offset"=0.0, "Gain"=1.0}, {"Color Box"=16711680, "Boolean"=FALSE, "List 2"=21, "Boolean 2"=FALSE, "Boolean 3"=FALSE, "Offset"=0.0, "Gain"=1.0}], "Gain Calculations"={"Threshold Trace"=1, "Min Thresh/%"=0.2, "Max Thresh/%"=0.8, "Gain calculated by dividing"=13, "Gain Range"=enum."Best Est", "Pre-peak-ms"=30.0, "by"=1}, "Impulse Plane"=enum."Yaw", "Impulse Direction"=FALSE}, {"Plot Traces"=[{"Color Box"=4652800, "Boolean"=TRUE, "List 2"=6, "Boolean 2"=TRUE, "Boolean 3"=FALSE, "Offset"=0.0, "Gain"=1.0}, {"Color Box"=1966335, "Boolean"=TRUE, "List 2"=12, "Boolean 2"=TRUE, "Boolean 3"=FALSE, "Offset"=0.0, "Gain"=1.0}, {"Color Box"=16722474, "Boolean"=FALSE, "List 2"=22, "Boolean 2"=FALSE, "Boolean 3"=FALSE, "Offset"=0.0, "Gain"=1.0}], "Gain Calculations"={"Threshold Trace"=6, "Min Thresh/%"=0.2, "Max Thresh/%"=0.8, "Gain calculated by dividing"=12, "Gain Range"=enum."Best Est", "Pre-peak-ms"=30.0, "by"=6}, "Impulse Plane"=enum."LARP", "Impulse Direction"=FALSE}, {"Plot Traces"=[{"Color Box"=4652800, "Boolean"=TRUE, "List 2"=7, "Boolean 2"=FALSE, "Boolean 3"=FALSE, "Offset"=0.0, "Gain"=1.0}, {"Color Box"=1966335, "Boolean"=TRUE, "List 2"=12, "Boolean 2"=TRUE, "Boolean 3"=FALSE, "Offset"=0.0, "Gain"=1.0}, {"Color Box"=16722474, "Boolean"=FALSE, "List 2"=23, "Boolean 2"=TRUE, "Boolean 3"=FALSE, "Offset"=0.0, "Gain"=1.0}], "Gain Calculations"={"Threshold Trace"=7, "Min Thresh/%"=0.2, "Max Thresh/%"=0.8, "Gain calculated by dividing"=12, "Gain Range"=enum."Best Est", "Pre-peak-ms"=30.0, "by"=7}, "Impulse Plane"=enum."RALP", "Impulse Direction"=TRUE}, {"Plot Traces"=[{"Color Box"=4652800, "Boolean"=TRUE, "List 2"=7, "Boolean 2"=TRUE, "Boolean 3"=FALSE, "Offset"=0.0, "Gain"=1.0}, {"Color Box"=1966335, "Boolean"=TRUE, "List 2"=12, "Boolean 2"=FALSE, "Boolean 3"=FALSE, "Offset"=0.0, "Gain"=1.0}, {"Color Box"=16722474, "Boolean"=FALSE, "List 2"=23, "Boolean 2"=FALSE, "Boolean 3"=FALSE, "Offset"=0.0, "Gain"=1.0}], "Gain Calculations"={"Threshold Trace"=7, "Min Thresh/%"=0.2, "Max Thresh/%"=0.8, "Gain calculated by dividing"=12, "Gain Range"=enum."Best Est", "Pre-peak-ms"=30.0, "by"=7}, "Impulse Plane"=enum."RALP", "Impulse Direction"=FALSE}, {"Plot Traces"=[{"Color Box"=4652800, "Boolean"=TRUE, "List 2"=6, "Boolean 2"=FALSE, "Boolean 3"=FALSE, "Offset"=0.0, "Gain"=1.0}, {"Color Box"=1966335, "Boolean"=TRUE, "List 2"=12, "Boolean 2"=FALSE, "Boolean 3"=FALSE, "Offset"=0.0, "Gain"=1.0}, {"Color Box"=16722474, "Boolean"=FALSE, "List 2"=22, "Boolean 2"=TRUE, "Boolean 3"=FALSE, "Offset"=0.0, "Gain"=1.0}], "Gain Calculations"={"Threshold Trace"=6, "Min Thresh/%"=0.2, "Max Thresh/%"=0.8, "Gain calculated by dividing"=12, "Gain Range"=enum."Best Est", "Pre-peak-ms"=30.0, "by"=6}, "Impulse Plane"=enum."LARP", "Impulse Direction"=TRUE}] ("Graph Properties")) -> ()  [unwired: 2 in, 2 out]
      }
      event "PS - EyHy": Value Change {
        # "Apply selected preset graph properties"
        n17 = event-data() -> ()  [unwired: 1 in, 6 out]
        n18 = property on="Graph Properties" class="Arr (strict)"("Val(Sgnl)"=T6 [{"Plot Traces"=[{"Color Box"=6618880, "Boolean"=TRUE, "List 2"=1, "Boolean 2"=FALSE, "Boolean 3"=FALSE, "Offset"=0.0, "Gain"=1.0}, {"Color Box"=4467455, "Boolean"=TRUE, "List 2"=13, "Boolean 2"=TRUE, "Boolean 3"=FALSE, "Offset"=0.0, "Gain"=1.0}, {"Color Box"=16711680, "Boolean"=FALSE, "List 2"=21, "Boolean 2"=TRUE, "Boolean 3"=FALSE, "Offset"=0.0, "Gain"=1.0}], "Gain Calculations"={"Threshold Trace"=1, "Min Thresh/%"=0.2, "Max Thresh/%"=0.8, "Gain calculated by dividing"=13, "Gain Range"=enum."Best Est", "Pre-peak-ms"=30.0, "by"=1}, "Impulse Plane"=enum."Yaw", "Impulse Direction"=TRUE}, {"Plot Traces"=[{"Color Box"=6618880, "Boolean"=TRUE, "List 2"=1, "Boolean 2"=TRUE, "Boolean 3"=FALSE, "Offset"=0.0, "Gain"=1.0}, {"Color Box"=1966335, "Boolean"=TRUE, "List 2"=13, "Boolean 2"=FALSE, "Boolean 3"=FALSE, "Offset"=0.0, "Gain"=1.0}, {"Color Box"=16711680, "Boolean"=FALSE, "List 2"=21, "Boolean 2"=FALSE, "Boolean 3"=FALSE, "Offset"=0.0, "Gain"=1.0}], "Gain Calculations"={"Threshold Trace"=1, "Min Thresh/%"=0.2, "Max Thresh/%"=0.8, "Gain calculated by dividing"=13, "Gain Range"=enum."Best Est", "Pre-peak-ms"=30.0, "by"=1}, "Impulse Plane"=enum."Yaw", "Impulse Direction"=FALSE}, {"Plot Traces"=[{"Color Box"=4652800, "Boolean"=TRUE, "List 2"=3, "Boolean 2"=FALSE, "Boolean 3"=FALSE, "Offset"=0.0, "Gain"=1.0}, {"Color Box"=1966335, "Boolean"=TRUE, "List 2"=12, "Boolean 2"=TRUE, "Boolean 3"=FALSE, "Offset"=0.0, "Gain"=1.0}, {"Color Box"=16722474, "Boolean"=FALSE, "List 2"=22, "Boolean 2"=FALSE, "Boolean 3"=FALSE, "Offset"=0.0, "Gain"=1.0}], "Gain Calculations"={"Threshold Trace"=3, "Min Thresh/%"=0.2, "Max Thresh/%"=0.8, "Gain calculated by dividing"=12, "Gain Range"=enum."Best Est", "Pre-peak-ms"=30.0, "by"=3}, "Impulse Plane"=enum."LARP", "Impulse Direction"=FALSE}, {"Plot Traces"=[{"Color Box"=4652800, "Boolean"=TRUE, "List 2"=3, "Boolean 2"=FALSE, "Boolean 3"=FALSE, "Offset"=0.0, "Gain"=1.0}, {"Color Box"=1966335, "Boolean"=TRUE, "List 2"=12, "Boolean 2"=TRUE, "Boolean 3"=FALSE, "Offset"=0.0, "Gain"=1.0}, {"Color Box"=16722474, "Boolean"=FALSE, "List 2"=23, "Boolean 2"=TRUE, "Boolean 3"=FALSE, "Offset"=0.0, "Gain"=1.0}], "Gain Calculations"={"Threshold Trace"=3, "Min Thresh/%"=0.2, "Max Thresh/%"=0.8, "Gain calculated by dividing"=12, "Gain Range"=enum."Best Est", "Pre-peak-ms"=30.0, "by"=3}, "Impulse Plane"=enum."RALP", "Impulse Direction"=TRUE}, {"Plot Traces"=[{"Color Box"=4652800, "Boolean"=TRUE, "List 2"=3, "Boolean 2"=TRUE, "Boolean 3"=FALSE, "Offset"=0.0, "Gain"=1.0}, {"Color Box"=1966335, "Boolean"=TRUE, "List 2"=12, "Boolean 2"=FALSE, "Boolean 3"=FALSE, "Offset"=0.0, "Gain"=1.0}, {"Color Box"=16722474, "Boolean"=FALSE, "List 2"=23, "Boolean 2"=FALSE, "Boolean 3"=FALSE, "Offset"=0.0, "Gain"=1.0}], "Gain Calculations"={"Threshold Trace"=3, "Min Thresh/%"=0.2, "Max Thresh/%"=0.8, "Gain calculated by dividing"=12, "Gain Range"=enum."Best Est", "Pre-peak-ms"=30.0, "by"=3}, "Impulse Plane"=enum."RALP", "Impulse Direction"=FALSE}, {"Plot Traces"=[{"Color Box"=4652800, "Boolean"=TRUE, "List 2"=3, "Boolean 2"=TRUE, "Boolean 3"=FALSE, "Offset"=0.0, "Gain"=1.0}, {"Color Box"=1966335, "Boolean"=TRUE, "List 2"=12, "Boolean 2"=FALSE, "Boolean 3"=FALSE, "Offset"=0.0, "Gain"=1.0}, {"Color Box"=16722474, "Boolean"=FALSE, "List 2"=22, "Boolean 2"=TRUE, "Boolean 3"=FALSE, "Offset"=0.0, "Gain"=1.0}], "Gain Calculations"={"Threshold Trace"=3, "Min Thresh/%"=0.2, "Max Thresh/%"=0.8, "Gain calculated by dividing"=12, "Gain Range"=enum."Best Est", "Pre-peak-ms"=30.0, "by"=3}, "Impulse Plane"=enum."LARP", "Impulse Direction"=TRUE}] ("Graph Properties")) -> ()  [unwired: 2 in, 2 out]
      }
      event "PS - RollPitch": Value Change {
        # "Apply selected preset graph properties"
        n19 = event-data() -> ()  [unwired: 1 in, 6 out]
        n20 = property on="Graph Properties" class="Arr (strict)"("Val(Sgnl)"=T6 [{"Plot Traces"=[{"Color Box"=6618880, "Boolean"=TRUE, "List 2"=1, "Boolean 2"=FALSE, "Boolean 3"=FALSE, "Offset"=0.0, "Gain"=1.0}, {"Color Box"=4467455, "Boolean"=TRUE, "List 2"=13, "Boolean 2"=TRUE, "Boolean 3"=FALSE, "Offset"=0.0, "Gain"=1.0}, {"Color Box"=16711680, "Boolean"=FALSE, "List 2"=21, "Boolean 2"=TRUE, "Boolean 3"=FALSE, "Offset"=0.0, "Gain"=1.0}], "Gain Calculations"={"Threshold Trace"=1, "Min Thresh/%"=0.2, "Max Thresh/%"=0.8, "Gain calculated by dividing"=13, "Gain Range"=enum."Best Est", "Pre-peak-ms"=30.0, "by"=1}, "Impulse Plane"=enum."Yaw", "Impulse Direction"=TRUE}, {"Plot Traces"=[{"Color Box"=6618880, "Boolean"=TRUE, "List 2"=1, "Boolean 2"=TRUE, "Boolean 3"=FALSE, "Offset"=0.0, "Gain"=1.0}, {"Color Box"=1966335, "Boolean"=TRUE, "List 2"=13, "Boolean 2"=FALSE, "Boolean 3"=FALSE, "Offset"=0.0, "Gain"=1.0}, {"Color Box"=16711680, "Boolean"=FALSE, "List 2"=21, "Boolean 2"=FALSE, "Boolean 3"=FALSE, "Offset"=0.0, "Gain"=1.0}], "Gain Calculations"={"Threshold Trace"=1, "Min Thresh/%"=0.2, "Max Thresh/%"=0.8, "Gain calculated by dividing"=13, "Gain Range"=enum."Best Est", "Pre-peak-ms"=30.0, "by"=1}, "Impulse Plane"=enum."Yaw", "Impulse Direction"=FALSE}, {"Plot Traces"=[{"Color Box"=4652800, "Boolean"=TRUE, "List 2"=3, "Boolean 2"=FALSE, "Boolean 3"=FALSE, "Offset"=0.0, "Gain"=1.0}, {"Color Box"=1966335, "Boolean"=TRUE, "List 2"=5, "Boolean 2"=TRUE, "Boolean 3"=FALSE, "Offset"=0.0, "Gain"=1.0}, {"Color Box"=16722474, "Boolean"=FALSE, "List 2"=22, "Boolean 2"=FALSE, "Boolean 3"=FALSE, "Offset"=0.0, "Gain"=1.0}], "Gain Calculations"={"Threshold Trace"=3, "Min Thresh/%"=0.2, "Max Thresh/%"=0.8, "Gain calculated by dividing"=5, "Gain Range"=enum."Best Est", "Pre-peak-ms"=30.0, "by"=3}, "Impulse Plane"=enum."LARP", "Impulse Direction"=FALSE}, {"Plot Traces"=[{"Color Box"=4652800, "Boolean"=TRUE, "List 2"=3, "Boolean 2"=FALSE, "Boolean 3"=FALSE, "Offset"=0.0, "Gain"=1.0}, {"Color Box"=1966335, "Boolean"=TRUE, "List 2"=5, "Boolean 2"=FALSE, "Boolean 3"=FALSE, "Offset"=0.0, "Gain"=1.0}, {"Color Box"=16722474, "Boolean"=FALSE, "List 2"=23, "Boolean 2"=TRUE, "Boolean 3"=FALSE, "Offset"=0.0, "Gain"=1.0}], "Gain Calculations"={"Threshold Trace"=3, "Min Thresh/%"=0.2, "Max Thresh/%"=0.8, "Gain calculated by dividing"=5, "Gain Range"=enum."Best Est", "Pre-peak-ms"=30.0, "by"=3}, "Impulse Plane"=enum."RALP", "Impulse Direction"=TRUE}, {"Plot Traces"=[{"Color Box"=4652800, "Boolean"=TRUE, "List 2"=3, "Boolean 2"=TRUE, "Boolean 3"=FALSE, "Offset"=0.0, "Gain"=1.0}, {"Color Box"=1966335, "Boolean"=TRUE, "List 2"=5, "Boolean 2"=TRUE, "Boolean 3"=FALSE, "Offset"=0.0, "Gain"=1.0}, {"Color Box"=16722474, "Boolean"=FALSE, "List 2"=23, "Boolean 2"=FALSE, "Boolean 3"=FALSE, "Offset"=0.0, "Gain"=1.0}], "Gain Calculations"={"Threshold Trace"=3, "Min Thresh/%"=0.2, "Max Thresh/%"=0.8, "Gain calculated by dividing"=5, "Gain Range"=enum."Best Est", "Pre-peak-ms"=30.0, "by"=3}, "Impulse Plane"=enum."RALP", "Impulse Direction"=FALSE}, {"Plot Traces"=[{"Color Box"=4652800, "Boolean"=TRUE, "List 2"=3, "Boolean 2"=TRUE, "Boolean 3"=FALSE, "Offset"=0.0, "Gain"=1.0}, {"Color Box"=1966335, "Boolean"=TRUE, "List 2"=5, "Boolean 2"=FALSE, "Boolean 3"=FALSE, "Offset"=0.0, "Gain"=1.0}, {"Color Box"=16722474, "Boolean"=FALSE, "List 2"=22, "Boolean 2"=TRUE, "Boolean 3"=FALSE, "Offset"=0.0, "Gain"=1.0}], "Gain Calculations"={"Threshold Trace"=3, "Min Thresh/%"=0.2, "Max Thresh/%"=0.8, "Gain calculated by dividing"=5, "Gain Range"=enum."Best Est", "Pre-peak-ms"=30.0, "by"=3}, "Impulse Plane"=enum."LARP", "Impulse Direction"=TRUE}] ("Graph Properties")) -> ()  [unwired: 2 in, 2 out]
      }
      event "print all": Mouse Up {
        w20 = T7[] [enum."Print All"] items=["Idle", "Initialize", "Quit", "Analyze", "Print All", "Print Horizontal", "Save Text File", "Save To Excel", "Save To Excel (legacy)"] ("element")
        # "Request all data report is printed."
        n21 = event-data() -> ()  [unwired: 1 in, 8 out]
        n22 = Enqueue Element(queue=w21, element=w20) -> ()  [unwired: 2 in, 3 out]
      }
      event "print horizontal": Mouse Up {
        w22 = T7[] [enum."Print Horizontal"] items=["Idle", "Initialize", "Quit", "Analyze", "Print All", "Print Horizontal", "Save Text File", "Save To Excel", "Save To Excel (legacy)"] ("element")
        # "Request horizontal data report is printed."
        n23 = event-data() -> ()  [unwired: 1 in, 8 out]
        n24 = Enqueue Element(queue=w23, element=w22) -> ()  [unwired: 2 in, 3 out]
      }
      event "Save to Excel": Mouse Up {
        w24 = T7[] [enum."Save To Excel"] items=["Idle", "Initialize", "Quit", "Analyze", "Print All", "Print Horizontal", "Save Text File", "Save To Excel", "Save To Excel (legacy)"] ("element")
        # "Request save data to excel."
        n25 = event-data() -> ()  [unwired: 1 in, 8 out]
        n26 = Enqueue Element(queue=w25, element=w24) -> ()  [unwired: 2 in, 3 out]
      }
      event "Save to Excel (legacy)": Mouse Up {
        w26 = T7[] [enum."Save To Excel (legacy)"] items=["Idle", "Initialize", "Quit", "Analyze", "Print All", "Print Horizontal", "Save Text File", "Save To Excel", "Save To Excel (legacy)"] ("element")
        # "Request save data to excel in the legacy format (single row)."
        n27 = event-data() -> ()  [unwired: 1 in, 8 out]
        n28 = Enqueue Element(queue=w27, element=w26) -> ()  [unwired: 2 in, 3 out]
      }
      event "Save to File": Mouse Up {
        w28 = T7[] [enum."Save Text File"] items=["Idle", "Initialize", "Quit", "Analyze", "Print All", "Print Horizontal", "Save Text File", "Save To Excel", "Save To Excel (legacy)"] ("element")
        # "Request save data as text to file"
        n29 = event-data() -> ()  [unwired: 1 in, 8 out]
        n30 = Enqueue Element(queue=w29, element=w28) -> ()  [unwired: 2 in, 3 out]
      }
    }
  }
  n31 = while {
    tunnel: w2 -> [w35]
    shift-right: [w30] -> w1
    shift-left: "Data In" -> [w31]
    stop <- w32 stop-if-true
    # "Main Loop"
    n32 = Dequeue Element(queue=w35) -> (queue out=w33:refnum<queue>, element=w34:T7[])  [unwired: 2 in, 2 out]
    n33 = for {
      tunnel: w34 -> [w39] mode=indexing
      tunnel: w33 -> [_]
      tunnel: [w38] -> w32
      shift-right: [w36] -> w30
      shift-left: w31 -> [w37]
      n34 = case shown="\"Save To Excel\"" w39 {
        tunnel: [_ _ TRUE _ _ _ _ _ _] -> w38
        tunnel: w37 -> [w40 w41 w52 w54 w248 w282 w311 w385 w441]
        tunnel: [w40 w41 w52 w54 w248 w282 w311 w383 w442] -> w36
        frame "Idle", Default {
          # "Do nothing."
        }
        frame "Initialize" {
          # "Initialize front panel data"
          # "Get printers"
          # "Initialize plugin."
          n35 = Unbundle By Name(w41) -> ("Data File.Channel List"=w44:string[], "Experiment Parameters 2.Subject"=w43:string, "Experiment Parameters.Stimulus"=w42:string)
          n36 = property on="Graph Properties" class="Arr (strict)"("Val(Sgnl)"=T6 [{"Plot Traces"=[{"Color Box"=6618880, "Boolean"=TRUE, "List 2"=1, "Boolean 2"=FALSE, "Boolean 3"=FALSE, "Offset"=0.0, "Gain"=1.0}, {"Color Box"=4467455, "Boolean"=TRUE, "List 2"=13, "Boolean 2"=TRUE, "Boolean 3"=FALSE, "Offset"=0.0, "Gain"=1.0}, {"Color Box"=16711680, "Boolean"=FALSE, "List 2"=21, "Boolean 2"=TRUE, "Boolean 3"=FALSE, "Offset"=0.0, "Gain"=1.0}], "Gain Calculations"={"Threshold Trace"=1, "Min Thresh/%"=0.2, "Max Thresh/%"=0.8, "Gain calculated by dividing"=13, "Gain Range"=enum."Best Est", "Pre-peak-ms"=30.0, "by"=1}, "Impulse Plane"=enum."Yaw", "Impulse Direction"=TRUE}, {"Plot Traces"=[{"Color Box"=6618880, "Boolean"=TRUE, "List 2"=1, "Boolean 2"=TRUE, "Boolean 3"=FALSE, "Offset"=0.0, "Gain"=1.0}, {"Color Box"=1966335, "Boolean"=TRUE, "List 2"=13, "Boolean 2"=FALSE, "Boolean 3"=FALSE, "Offset"=0.0, "Gain"=1.0}, {"Color Box"=16711680, "Boolean"=FALSE, "List 2"=21, "Boolean 2"=FALSE, "Boolean 3"=FALSE, "Offset"=0.0, "Gain"=1.0}], "Gain Calculations"={"Threshold Trace"=1, "Min Thresh/%"=0.2, "Max Thresh/%"=0.8, "Gain calculated by dividing"=13, "Gain Range"=enum."Best Est", "Pre-peak-ms"=30.0, "by"=1}, "Impulse Plane"=enum."Yaw", "Impulse Direction"=FALSE}, {"Plot Traces"=[{"Color Box"=4652800, "Boolean"=TRUE, "List 2"=6, "Boolean 2"=TRUE, "Boolean 3"=FALSE, "Offset"=0.0, "Gain"=1.0}, {"Color Box"=1966335, "Boolean"=TRUE, "List 2"=14, "Boolean 2"=FALSE, "Boolean 3"=FALSE, "Offset"=0.0, "Gain"=1.0}, {"Color Box"=16722474, "Boolean"=FALSE, "List 2"=22, "Boolean 2"=FALSE, "Boolean 3"=FALSE, "Offset"=0.0, "Gain"=1.0}], "Gain Calculations"={"Threshold Trace"=6, "Min Thresh/%"=0.2, "Max Thresh/%"=0.8, "Gain calculated by dividing"=14, "Gain Range"=enum."Best Est", "Pre-peak-ms"=30.0, "by"=6}, "Impulse Plane"=enum."LARP", "Impulse Direction"=FALSE}, {"Plot Traces"=[{"Color Box"=4652800, "Boolean"=TRUE, "List 2"=7, "Boolean 2"=FALSE, "Boolean 3"=FALSE, "Offset"=0.0, "Gain"=1.0}, {"Color Box"=1966335, "Boolean"=TRUE, "List 2"=15, "Boolean 2"=TRUE, "Boolean 3"=FALSE, "Offset"=0.0, "Gain"=1.0}, {"Color Box"=16722474, "Boolean"=FALSE, "List 2"=23, "Boolean 2"=TRUE, "Boolean 3"=FALSE, "Offset"=0.0, "Gain"=1.0}], "Gain Calculations"={"Threshold Trace"=7, "Min Thresh/%"=0.2, "Max Thresh/%"=0.8, "Gain calculated by dividing"=15, "Gain Range"=enum."Best Est", "Pre-peak-ms"=30.0, "by"=7}, "Impulse Plane"=enum."RALP", "Impulse Direction"=TRUE}, {"Plot Traces"=[{"Color Box"=4652800, "Boolean"=TRUE, "List 2"=7, "Boolean 2"=TRUE, "Boolean 3"=FALSE, "Offset"=0.0, "Gain"=1.0}, {"Color Box"=1966335, "Boolean"=TRUE, "List 2"=15, "Boolean 2"=FALSE, "Boolean 3"=FALSE, "Offset"=0.0, "Gain"=1.0}, {"Color Box"=16722474, "Boolean"=FALSE, "List 2"=23, "Boolean 2"=FALSE, "Boolean 3"=FALSE, "Offset"=0.0, "Gain"=1.0}], "Gain Calculations"={"Threshold Trace"=7, "Min Thresh/%"=0.2, "Max Thresh/%"=0.8, "Gain calculated by dividing"=15, "Gain Range"=enum."Best Est", "Pre-peak-ms"=30.0, "by"=7}, "Impulse Plane"=enum."RALP", "Impulse Direction"=FALSE}, {"Plot Traces"=[{"Color Box"=4652800, "Boolean"=TRUE, "List 2"=6, "Boolean 2"=FALSE, "Boolean 3"=FALSE, "Offset"=0.0, "Gain"=1.0}, {"Color Box"=1966335, "Boolean"=TRUE, "List 2"=14, "Boolean 2"=TRUE, "Boolean 3"=FALSE, "Offset"=0.0, "Gain"=1.0}, {"Color Box"=16722474, "Boolean"=FALSE, "List 2"=22, "Boolean 2"=TRUE, "Boolean 3"=FALSE, "Offset"=0.0, "Gain"=1.0}], "Gain Calculations"={"Threshold Trace"=6, "Min Thresh/%"=0.2, "Max Thresh/%"=0.8, "Gain calculated by dividing"=14, "Gain Range"=enum."Best Est", "Pre-peak-ms"=30.0, "by"=6}, "Impulse Plane"=enum."LARP", "Impulse Direction"=TRUE}] ("Graph Properties")) -> ()  [unwired: 2 in, 2 out]
          n37 = property on="List 2" class="Ring (strict)"("Strings []"=w44) -> ()  [unwired: 2 in, 2 out]
          n38 = property on="by" class="Ring (strict)"("Strings []"=w44) -> ()  [unwired: 2 in, 2 out]
          n39 = property on="Gain calculated by dividing" class="Ring (strict)"("Strings []"=w44) -> ()  [unwired: 2 in, 2 out]
          n40 = property on="Threshold Trace" class="Ring (strict)"("Strings []"=w44) -> ()  [unwired: 2 in, 2 out]
          n41 = local write "Stimulus"(w42) -> ()
          n42 = local write "Patient ID"(w43) -> ()
          n43 = property on="Printer Select" class="CmbBox"("Value"="Retrieving available printers") -> (error out=w47:errorcluster)  [unwired: 2 in, 1 out]
          n44 = call <vilib>:"Query Available Printers.vi"("error in (no error)"=w47) -> ("error out"=w50:errorcluster, "default printer"=w48:string, "system configured printers"=w51:string[])  [unwired: 8 in]
          n45 = property on="Printer Select" class="CmbBox"(error in=w50, "Strings[]"=w51) -> (error out=w49:errorcluster)  [unwired: 1 in, 1 out]
          n46 = property on="Printer Select" class="CmbBox"(error in=w49, "Value"=w48) -> ()  [unwired: 1 in, 2 out]
        }
        frame "Quit" {
          # "End plugin execution."
        }
        frame "Analyze" {
          # "TODO: This was copied directly from the old implementation. Tidy it up."
          # "Do impulse analysis."
          n47 = local read "Impulse Gain Method"() -> (w60:T5)
          n48 = local read "Impulse Group Gain Method"() -> (w61:T4)
          n49 = local read "Graph Properties"() -> (w62:T6)
          n50 = Unbundle By Name(w54) -> ("desacc"=w65:T12, "Data File"=w64:T13, "Impulse Positions"=w63:T14, "Data File.Sample Rate"=w56:i32)
          n51 = To Double Precision Float(number=w56) -> (double precision float=w57:dbl)
          n52 = Bundle("Impulse Gain Method"=w60, "Impulse Group Gain Method"=w61) -> (w59:T15)  [unwired: 1 in]
          n53 = Divide(x=1000.0 ("y"), y=w57) -> (x/y=w55:dbl)
          n54 = for {
            tunnel: w62 -> [w74] mode=indexing
            tunnel: w63 -> [w79]
            tunnel: w64 -> [w78]
            tunnel: w55 -> [w73]
            tunnel: w56 -> [w69]
            tunnel: w59 -> [w67]
            tunnel: w65 -> [w66]
            i -> [w70]
            n55 = Unbundle By Name(w74) -> ("Impulse Direction"=w71:bool, "Impulse Plane"=w72:T16, "Plot Traces"=w75:T17)
            n56 = call "Couple Head Impulse Traces.vi"("Data Input"=w78, "Impulse Positions"=w79, "Impulse Direction +ve?"=w71, "Impulse Plane"=w72, "Plot Selection 2"=w75, "desacc"=w66, "Interpolate"=TRUE) -> ("No Impulses"=w76:i32, "Impulses"=w77:dbl[][])  [unwired: 9 in, 2 out]
            n57 = case shown="0, Default" w70 {
              tunnel: w77 -> [w88 w116 w144 w172 w200 w228]
              tunnel: w76 -> [w90 w118 w146 w174 w202 w230]
              tunnel: w75 -> [w87 w115 w143 w171 w199 w227]
              tunnel: w74 -> [w89 w117 w145 w173 w201 w229]
              tunnel: w73 -> [w91 w119 w147 w175 w203 w231]
              tunnel: w69 -> [w92 w120 w148 w176 w204 w232]
              tunnel: w67 -> [w86 w114 w142 w170 w198 w226]
              frame 0, Default {
                n58 = Bundle(0.0, w91, "Impulses"=w88) -> (w85:cluster{dbl, dbl, "Impulses":dbl[][]})  [unwired: 1 in]
                n59 = for {
                  tunnel: w87 -> [w99] mode=indexing
                  tunnel: w90 -> [w96]
                  i -> [w97]
                  n60 = Unbundle By Name(w99) -> ("Color Box"=w98:u32, "Boolean"=w94:bool)
                  n61 = Multiply(x=w96, y=w97) -> (x*y=w95:i32)
                  n62 = for {
                    N: w96 -> [_]
                    tunnel: w98 -> [w101]
                    tunnel: w95 -> [w104]
                    tunnel: w94 -> [w102]
                    i -> [w103]
                    n63 = Add(x=w104, y=w103) -> (x+y=w100:i32)
                    n64 = stacked-sequence {
                      tunnel: w101 -> [_ w107]
                      tunnel: w100 -> [w105 _]
                      tunnel: w102 -> [_ w106]
                      frame #0 {
                        n65 = property on="0" class="WFGraph (strict)"("Active Plot"=w105) -> ()  [unwired: 2 in, 2 out]
                      }
                      frame #1 {
                        n66 = property on="0" class="WFGraph (strict)"("Plot.Plot Color"=w107, "Plot.Visible"=w106) -> ()  [unwired: 2 in, 2 out]
                      }
                    }
                  }
                }
                n67 = call "Gain.vi"("Sample Rate"=w92, "Number of Impulses"=w90, "Graph Cluster"=w89, "Gain Methods"=w86, "Data (in)"=w88) -> ("STD"=w83:dbl, "sd peak vel"=w80:dbl, "N"=w82:i32, "GAIN"=w84:dbl, "mean peak vel"=w81:dbl)
                n68 = local write "0"(w85) -> ()
                n69 = local write "0 N"(w82) -> ()
                n70 = local write "0 Gain"(w84) -> ()
                n71 = local write "0 SD"(w83) -> ()
                n72 = local write "0 PeakVel"(w81) -> ()
                n73 = local write "0 PeakVel SD"(w80) -> ()
              }
              frame 1 {
                n74 = Bundle(0.0, w119, "Impulses"=w116) -> (w113:cluster{dbl, dbl, "Impulses":dbl[][]})  [unwired: 1 in]
                n75 = for {
                  tunnel: w115 -> [w127] mode=indexing
                  tunnel: w118 -> [w124]
                  i -> [w125]
                  n76 = Unbundle By Name(w127) -> ("Color Box"=w126:u32, "Boolean"=w122:bool)
                  n77 = Multiply(x=w124, y=w125) -> (x*y=w123:i32)
                  n78 = for {
                    N: w124 -> [_]
                    tunnel: w126 -> [w132]
                    tunnel: w123 -> [w131]
                    tunnel: w122 -> [w128]
                    i -> [w130]
                    n79 = Add(x=w131, y=w130) -> (x+y=w129:i32)
                    n80 = stacked-sequence {
                      tunnel: w132 -> [_ w135]
                      tunnel: w129 -> [w133 _]
                      tunnel: w128 -> [_ w134]
                      frame #0 {
                        n81 = property on="1" class="WFGraph (strict)"("Active Plot"=w133) -> ()  [unwired: 2 in, 2 out]
                      }
                      frame #1 {
                        n82 = property on="1" class="WFGraph (strict)"("Plot.Plot Color"=w135, "Plot.Visible"=w134) -> ()  [unwired: 2 in, 2 out]
                      }
                    }
                  }
                }
                n83 = call "Gain.vi"("Sample Rate"=w120, "Number of Impulses"=w118, "Graph Cluster"=w117, "Gain Methods"=w114, "Data (in)"=w116) -> ("STD"=w111:dbl, "sd peak vel"=w108:dbl, "N"=w110:i32, "GAIN"=w112:dbl, "mean peak vel"=w109:dbl)
                n84 = local write "1"(w113) -> ()
                n85 = local write "1 Gain"(w112) -> ()
                n86 = local write "1 N"(w110) -> ()
                n87 = local write "1 SD"(w111) -> ()
                n88 = local write "1 PeakVel"(w109) -> ()
                n89 = local write "1 PeakVel SD"(w108) -> ()
              }
              frame 2 {
                n90 = Bundle(0.0, w147, "Impulses"=w144) -> (w141:cluster{dbl, dbl, "Impulses":dbl[][]})  [unwired: 1 in]
                n91 = for {
                  tunnel: w143 -> [w155] mode=indexing
                  tunnel: w146 -> [w152]
                  i -> [w153]
                  n92 = Unbundle By Name(w155) -> ("Color Box"=w154:u32, "Boolean"=w150:bool)
                  n93 = Multiply(x=w152, y=w153) -> (x*y=w151:i32)
                  n94 = for {
                    N: w152 -> [_]
                    tunnel: w154 -> [w158]
                    tunnel: w151 -> [w160]
                    tunnel: w150 -> [w157]
                    i -> [w159]
                    n95 = Add(x=w160, y=w159) -> (x+y=w156:i32)
                    n96 = stacked-sequence {
                      tunnel: w158 -> [_ w163]
                      tunnel: w156 -> [w161 _]
                      tunnel: w157 -> [_ w162]
                      frame #0 {
                        n97 = property on="2" class="WFGraph (strict)"("Active Plot"=w161) -> ()  [unwired: 2 in, 2 out]
                      }
                      frame #1 {
                        n98 = property on="2" class="WFGraph (strict)"("Plot.Plot Color"=w163, "Plot.Visible"=w162) -> ()  [unwired: 2 in, 2 out]
                      }
                    }
                  }
                }
                n99 = call "Gain.vi"("Sample Rate"=w148, "Number of Impulses"=w146, "Graph Cluster"=w145, "Gain Methods"=w142, "Data (in)"=w144) -> ("STD"=w139:dbl, "sd peak vel"=w136:dbl, "N"=w138:i32, "GAIN"=w140:dbl, "mean peak vel"=w137:dbl)
                n100 = local write "2"(w141) -> ()
                n101 = local write "2 Gain"(w140) -> ()
                n102 = local write "2 N"(w138) -> ()
                n103 = local write "2 SD"(w139) -> ()
                n104 = local write "2 PeakVel"(w137) -> ()
                n105 = local write "2 PeakVel SD"(w136) -> ()
              }
              frame 3 {
                n106 = Bundle(0.0, w175, "Impulses"=w172) -> (w169:cluster{dbl, dbl, "Impulses":dbl[][]})  [unwired: 1 in]
                n107 = for {
                  tunnel: w171 -> [w183] mode=indexing
                  tunnel: w174 -> [w180]
                  i -> [w181]
                  n108 = Unbundle By Name(w183) -> ("Color Box"=w182:u32, "Boolean"=w178:bool)
                  n109 = Multiply(x=w180, y=w181) -> (x*y=w179:i32)
                  n110 = for {
                    N: w180 -> [_]
                    tunnel: w182 -> [w185]
                    tunnel: w179 -> [w188]
                    tunnel: w178 -> [w186]
                    i -> [w187]
                    n111 = Add(x=w188, y=w187) -> (x+y=w184:i32)
                    n112 = stacked-sequence {
                      tunnel: w185 -> [_ w191]
                      tunnel: w184 -> [w189 _]
                      tunnel: w186 -> [_ w190]
                      frame #0 {
                        n113 = property on="3" class="WFGraph (strict)"("Active Plot"=w189) -> ()  [unwired: 2 in, 2 out]
                      }
                      frame #1 {
                        n114 = property on="3" class="WFGraph (strict)"("Plot.Plot Color"=w191, "Plot.Visible"=w190) -> ()  [unwired: 2 in, 2 out]
                      }
                    }
                  }
                }
                n115 = call "Gain.vi"("Sample Rate"=w176, "Number of Impulses"=w174, "Graph Cluster"=w173, "Gain Methods"=w170, "Data (in)"=w172) -> ("STD"=w167:dbl, "sd peak vel"=w164:dbl, "N"=w166:i32, "GAIN"=w168:dbl, "mean peak vel"=w165:dbl)
                n116 = local write "3"(w169) -> ()
                n117 = local write "3 N"(w166) -> ()
                n118 = local write "3 Gain"(w168) -> ()
                n119 = local write "3 SD"(w167) -> ()
                n120 = local write "3 PeakVel"(w165) -> ()
                n121 = local write "3 PeakVel SD"(w164) -> ()
              }
              frame 4 {
                n122 = Bundle(0.0, w203, "Impulses"=w200) -> (w197:cluster{dbl, dbl, "Impulses":dbl[][]})  [unwired: 1 in]
                n123 = for {
                  tunnel: w199 -> [w211] mode=indexing
                  tunnel: w202 -> [w208]
                  i -> [w209]
                  n124 = Unbundle By Name(w211) -> ("Color Box"=w210:u32, "Boolean"=w206:bool)
                  n125 = Multiply(x=w208, y=w209) -> (x*y=w207:i32)
                  n126 = for {
                    N: w208 -> [_]
                    tunnel: w210 -> [w214]
                    tunnel: w207 -> [w216]
                    tunnel: w206 -> [w213]
                    i -> [w215]
                    n127 = Add(x=w216, y=w215) -> (x+y=w212:i32)
                    n128 = stacked-sequence {
                      tunnel: w214 -> [_ w219]
                      tunnel: w212 -> [w217 _]
                      tunnel: w213 -> [_ w218]
                      frame #0 {
                        n129 = property on="4" class="WFGraph (strict)"("Active Plot"=w217) -> ()  [unwired: 2 in, 2 out]
                      }
                      frame #1 {
                        n130 = property on="4" class="WFGraph (strict)"("Plot.Plot Color"=w219, "Plot.Visible"=w218) -> ()  [unwired: 2 in, 2 out]
                      }
                    }
                  }
                }
                n131 = call "Gain.vi"("Sample Rate"=w204, "Number of Impulses"=w202, "Graph Cluster"=w201, "Gain Methods"=w198, "Data (in)"=w200) -> ("STD"=w195:dbl, "sd peak vel"=w192:dbl, "N"=w194:i32, "GAIN"=w196:dbl, "mean peak vel"=w193:dbl)
                n132 = local write "4 Gain"(w196) -> ()
                n133 = local write "4 N"(w194) -> ()
                n134 = local write "4"(w197) -> ()
                n135 = local write "4 SD"(w195) -> ()
                n136 = local write "4 PeakVel"(w193) -> ()
                n137 = local write "4 PeakVel SD"(w192) -> ()
              }
              frame 5 {
                n138 = Bundle(0.0, w231, "Impulses"=w228) -> (w225:cluster{dbl, dbl, "Impulses":dbl[][]})  [unwired: 1 in]
                n139 = for {
                  tunnel: w227 -> [w239] mode=indexing
                  tunnel: w230 -> [w236]
                  i -> [w237]
                  n140 = Unbundle By Name(w239) -> ("Color Box"=w238:u32, "Boolean"=w234:bool)
                  n141 = Multiply(x=w236, y=w237) -> (x*y=w235:i32)
                  n142 = for {
                    N: w236 -> [_]
                    tunnel: w238 -> [w241]
                    tunnel: w235 -> [w244]
                    tunnel: w234 -> [w242]
                    i -> [w243]
                    n143 = Add(x=w244, y=w243) -> (x+y=w240:i32)
                    n144 = stacked-sequence {
                      tunnel: w241 -> [_ w247]
                      tunnel: w240 -> [w245 _]
                      tunnel: w242 -> [_ w246]
                      frame #0 {
                        n145 = property on="5" class="WFGraph (strict)"("Active Plot"=w245) -> ()  [unwired: 2 in, 2 out]
                      }
                      frame #1 {
                        n146 = property on="5" class="WFGraph (strict)"("Plot.Plot Color"=w247, "Plot.Visible"=w246) -> ()  [unwired: 2 in, 2 out]
                      }
                    }
                  }
                }
                n147 = call "Gain.vi"("Sample Rate"=w232, "Number of Impulses"=w230, "Graph Cluster"=w229, "Gain Methods"=w226, "Data (in)"=w228) -> ("STD"=w223:dbl, "sd peak vel"=w220:dbl, "N"=w222:i32, "GAIN"=w224:dbl, "mean peak vel"=w221:dbl)
                n148 = local write "5"(w225) -> ()
                n149 = local write "5 N"(w222) -> ()
                n150 = local write "5 Gain"(w224) -> ()
                n151 = local write "5 SD"(w223) -> ()
                n152 = local write "5 PeakVel"(w221) -> ()
                n153 = local write "5 PeakVel SD"(w220) -> ()
              }
            }
          }
        }
        frame "Print All" {
          # "Unfortunately the report functions do not accept\npicture data. In order to print this image a temporary\nfile is made in the application directory."
          # "The get front panel image vi function currently does not work with splitter panes. This code works around this issue by:\n1. Expanding the front panel so that all controls are visible\n2. Getting an image of the expanded panel.\n3. Resizing the front panel back to normal.\n4. Extracting the picture region which contains the top pane controls.\n5. Printing the extracted image."
          # "Print a report of all canals."
          n154 = call <userlib>:"Current VIs Reference__ogtk.vi"() -> ("Current VI's reference"=w249:refnum<vi>)  [unwired: 5 in]
          n155 = control-ref of="Splitter"() -> (w273:refnum<vi>)
          n156 = property class="VI"(reference=w249) -> (reference out=w250:refnum<vi>, error out=w251:errorcluster, "Front Panel.PanelBounds"=w255:T10)  [unwired: 1 in]
          n157 = property class="VI"(reference=w250, error in=w251, "Front Panel.PanelBounds"=T10 {"Left"=0, "Top"=0, "Right"=900, "Bottom"=1250} ("Front Panel Window:Panel Bounds")) -> (reference out=w253:refnum<vi>, error out=w252:errorcluster)
          n158 = invoke class="VI" method="FP.Get Image"(reference=w253, error in=w252, "visible area only"=FALSE ("Visible Area Only")) -> (reference out=w254:refnum<vi>, error out=w275:errorcluster, "image data"=w263:T18)  [unwired: 3 in, 3 out]
          n159 = property class="Splitter"(reference=w273, error in=w275) -> (error out=w276:errorcluster, "Position"=w274:i32)  [unwired: 1 out]
          n160 = Bundle By Name(cluster=T9 {"left"=0, "top"=0, "right"=0, "bottom"=0} ("subset rect"), "left"=i16 0, "top"=i16 0, "right"=i16 900, "bottom"=w274) -> (w259:T9)
          n161 = call <vilib>:"Get Image Subset.vi"("subset rect"=w259, "image data"=w263) -> ("image subset"=w279:T18)  [unwired: 4 in, 1 out]
          n162 = call <userlib>:"Application Directory__ogtk.vi"() -> ("Application Directory (+ Relative)"=w277:path)  [unwired: 1 in]
          n163 = Build Path(base path=w277, name or relative path="temp.png") -> (appended path=w280:path)
          n164 = call <vilib>:"Write JPEG File.vi"("image data"=w279, "path to JPEG file"=w280) -> ("error out"=w281:errorcluster)  [unwired: 8 in, 1 out]
          n165 = call <vilib>:"New Report.vi"("report type"=T8."Standard Report", "error in (no error)"=w281) -> ("report out"=w264:refnum<class "NI_report.lvclass">, "error out"=w265:errorcluster)  [unwired: 12 in]
          n166 = property on="Printer Select" class="CmbBox"() -> ("Value"=w270:string)  [unwired: 2 in, 2 out]
          n167 = call-poly <vilib>:"Append Image to Report.vi"("report in"=w264, "path or URL of image"=w280, "error in (no error)"=w265) -> ("report out"=w267:refnum<class "NI_report.lvclass">, "error out"=w268:errorcluster)  [unwired: 9 in, 2 out]
          n168 = call-dynamic "Print Report.vi"("report in"=w267, "printer name (default)"=w270, "error in (no error)"=w268) -> ("report out"=w266:refnum<class "NI_report.lvclass">, "error out"=w269:errorcluster)  [unwired: 11 in]
          n169 = property class="VI"(reference=w254, error in=w276, "Front Panel.PanelBounds"=w255) -> ()  [unwired: 2 out]
          n170 = call-dynamic "Dispose Report.vi"("report in"=w266, "error in (no error)"=w269) -> ("error out"=w271:errorcluster)  [unwired: 13 in]
          n171 = Delete(path (use dialog)=w280, error in=w271) -> ()  [unwired: 3 in, 3 out]
        }
        frame "Print Horizontal" {
          w299 = "Standard Deviation"
          w298 = "Gain"
          # "Generate headings and \ncontrol references"
          # "Print and close \nreport."
          # "Put listed controls and\nheadings in report."
          # "Make new report."
          # "Print a report of horizontal canals."
          n172 = control-ref of="0"() -> (w285:refnum<vi>)
          n173 = control-ref of="0 Gain"() -> (w290:refnum<vi>)
          n174 = control-ref of="0 SD"() -> (w291:refnum<vi>)
          n175 = control-ref of="1"() -> (w292:refnum<vi>)
          n176 = control-ref of="1 Gain"() -> (w293:refnum<vi>)
          n177 = control-ref of="1 SD"() -> (w294:refnum<vi>)
          n178 = Build Array("---Horizontal Left---", w298, w299, "---Horizontal Right---", w298, w299) -> (w300:string[])
          n179 = Build Array(w285, w290, w291, w292, w293, w294) -> (w286:refnum<vi>[])
          n180 = call <vilib>:"New Report.vi"("report type"=T8."Standard Report") -> ("report out"=w301:refnum<class "NI_report.lvclass">, "error out"=w302:errorcluster)  [unwired: 13 in]
          n181 = for {
            shift-right: [w310] -> w287
            shift-left: w301 -> [w305]
            tunnel: w286 -> [w309] mode=indexing
            shift-right: [w308] -> w288
            shift-left: w302 -> [w304]
            tunnel: w300 -> [w303] mode=indexing
            n182 = call-poly <vilib>:"Append Report Text.vi"("report in"=w305, "text"=w303, "error in (no error)"=w304) -> ("report out"=w306:refnum<class "NI_report.lvclass">, "error out"=w307:errorcluster)  [unwired: 9 in, 2 out]
            n183 = call-dynamic "Append Control Image to Report.vi"("report in"=w306, "ctrl reference"=w309, "error in (no error)"=w307) -> ("report out"=w310:refnum<class "NI_report.lvclass">, "error out"=w308:errorcluster)  [unwired: 9 in, 2 out]
          }
          n184 = property on="Printer Select" class="CmbBox"() -> ("Value"=w295:string)  [unwired: 2 in, 2 out]
          n185 = call-dynamic "Print Report.vi"("report in"=w287, "printer name (default)"=w295, "error in (no error)"=w288) -> ("report out"=w283:refnum<class "NI_report.lvclass">, "error out"=w284:errorcluster)  [unwired: 11 in]
          n186 = call-dynamic "Dispose Report.vi"("report in"=w283, "error in (no error)"=w284) -> ()  [unwired: 13 in, 1 out]
        }
        frame "Save Text File" {
          # "Save results to a file as text."
          n187 = Open/Create/Replace File(prompt="Select File to Create or Append", operation (0:open)=T11."open or create") -> (refnum out=w314:refnum<file>, cancelled=w312:bool, error out=w313:errorcluster)  [unwired: 4 in]
          n188 = case shown="False" w312 {
            tunnel: w314 -> [w360 _]
            tunnel: w313 -> [w359 _]
            frame False {
              # "Operation not cancelled -> save data to file."
              n189 = Read from Text File(file (use dialog)=w360, error in=w359) -> (refnum out=w318:refnum<file>, text=w361:string, error out=w322:errorcluster)  [unwired: 2 in, 1 out]
              n190 = Equal?(x="", y=w361) -> (x = y?=w345:bool)
              n191 = Build Array("Subject Name", "LH Gain", "LH SD", "RH Gain", "RH SD", "LA Gain", "LA SD", "RA Gain", "RA SD", "LP Gain", "LP SD", "RP Gain", "RP SD") -> (w323:string[])
              n192 = Array To Spreadsheet String(array=w323, 3:"%s" ("format string")) -> (spreadsheet string=w320:string)  [unwired: 1 in]
              n193 = case shown="True" w345 {
                tunnel: [w362 w365] -> w327
                tunnel: w322 -> [w363 w368]
                tunnel: [w363 w367] -> w321
                tunnel: w320 -> [_ w366]
                tunnel: w318 -> [w362 w364]
                frame False {
                }
                frame True {
                  n194 = Write to Text File(file (use dialog)=w364, text=w366, error in=w368) -> (refnum out=w365:refnum<file>, error out=w367:errorcluster)  [unwired: 1 in, 1 out]
                }
              }
              n195 = local read "0 Gain"() -> (w343:dbl)
              n196 = local read "1 Gain"() -> (w341:dbl)
              n197 = local read "2 Gain"() -> (w339:dbl)
              n198 = local read "3 Gain"() -> (w337:dbl)
              n199 = local read "4 Gain"() -> (w335:dbl)
              n200 = local read "5 Gain"() -> (w333:dbl)
              n201 = local read "0 SD"() -> (w342:dbl)
              n202 = local read "1 SD"() -> (w340:dbl)
              n203 = local read "2 SD"() -> (w338:dbl)
              n204 = local read "3 SD"() -> (w336:dbl)
              n205 = local read "4 SD"() -> (w334:dbl)
              n206 = local read "5 SD"() -> (w332:dbl)
              n207 = Build Array(w343, w342, w341, w340, w339, w338, w337, w336, w335, w334, w333, w332) -> (w329:dbl[])
              n208 = local read "Patient ID"() -> (w317:string)
              n209 = Array To Spreadsheet String(array=w329, 3:"%.2f" ("format string")) -> (spreadsheet string=w331:string)  [unwired: 1 in]
              n210 = Concatenate Strings(w317, "\t", w331) -> (w326:string)
              n211 = Write to Text File(file (use dialog)=w327, text=w326, error in=w321) -> (refnum out=w324:refnum<file>, error out=w325:errorcluster)  [unwired: 1 in, 1 out]
              n212 = Close File(refnum=w324, error in=w325) -> ()  [unwired: 2 out]
            }
            frame True {
              # "Operation cancelled -> do nothing."
            }
          }
        }
        frame "Save To Excel" {
          w389 = string[] ["Patient ID", "Stimulus", "Impulse Gain Method", "Impulse Group Method", "Direction", "Gain", "SD", "n", "Peak Velocity", "Peak Velocity SD"]  # Header
          # "Build rows per impulse direction"
          # "Common row data"
          # "Save data to excel (row per impulse direction)."
          n213 = Unbundle By Name(w385) -> ("Excel"=w386:refnum<class "Excel.lvclass">)
          n214 = Unbundle By Name(w385) -> ("Experiment Parameters.Stimulus"=w422:string)
          n215 = property on="Impulse Gain Method" class="Enum (strict)"() -> ("Strings []"=w424:string[], "Value"=w426:T5)  [unwired: 2 in, 2 out]
          n216 = property on="Impulse Group Gain Method" class="Enum (strict)"() -> ("Strings []"=w425:string[], "Value"=w427:T4)  [unwired: 2 in, 2 out]
          n217 = local read "Patient ID"() -> (w423:string)
          n218 = Index Array(array=w424, index=w426) -> (element=w421:string)
          n219 = Index Array(array=w425, index=w427) -> (element=w420:string)
          n220 = Build Array(w423, w422, w421, w420) -> (w419:string[])
          n221 = local read "0 Gain"() -> (w418:dbl)
          n222 = local read "1 Gain"() -> (w417:dbl)
          n223 = local read "2 Gain"() -> (w416:dbl)
          n224 = local read "3 Gain"() -> (w415:dbl)
          n225 = local read "4 Gain"() -> (w414:dbl)
          n226 = local read "5 Gain"() -> (w413:dbl)
          n227 = local read "0 SD"() -> (w407:dbl)
          n228 = local read "1 SD"() -> (w408:dbl)
          n229 = local read "2 SD"() -> (w409:dbl)
          n230 = local read "3 SD"() -> (w410:dbl)
          n231 = local read "4 SD"() -> (w411:dbl)
          n232 = local read "5 SD"() -> (w412:dbl)
          n233 = local read "0 N"() -> (w401:i32)
          n234 = local read "1 N"() -> (w406:i32)
          n235 = local read "2 N"() -> (w405:i32)
          n236 = local read "3 N"() -> (w404:i32)
          n237 = local read "4 N"() -> (w403:i32)
          n238 = local read "5 N"() -> (w402:i32)
          n239 = Build Array(w418, w417, w416, w415, w414, w413) -> (w400:dbl[])
          n240 = Build Array(w407, w408, w409, w410, w411, w412) -> (w399:dbl[])
          n241 = Build Array(w401, w406, w405, w404, w403, w402) -> (w398:i32[])
          n242 = local read "0 PeakVel SD"() -> (w370:dbl)
          n243 = local read "1 PeakVel SD"() -> (w371:dbl)
          n244 = local read "2 PeakVel SD"() -> (w372:dbl)
          n245 = local read "3 PeakVel SD"() -> (w373:dbl)
          n246 = local read "4 PeakVel SD"() -> (w374:dbl)
          n247 = local read "5 PeakVel SD"() -> (w375:dbl)
          n248 = local read "0 PeakVel"() -> (w382:dbl)
          n249 = local read "1 PeakVel"() -> (w381:dbl)
          n250 = local read "2 PeakVel"() -> (w380:dbl)
          n251 = local read "3 PeakVel"() -> (w379:dbl)
          n252 = local read "4 PeakVel"() -> (w378:dbl)
          n253 = local read "5 PeakVel"() -> (w377:dbl)
          n254 = Build Array(w382, w381, w380, w379, w378, w377) -> (w376:dbl[])
          n255 = Build Array(w370, w371, w372, w373, w374, w375) -> (w369:dbl[])
          n256 = for {
            tunnel: w419 -> [w433]
            tunnel: [w437] -> w388 mode=indexing
            tunnel: w400 -> [w436] mode=indexing
            tunnel: w399 -> [w435] mode=indexing
            tunnel: w398 -> [w434] mode=indexing
            tunnel: string[] ["Left", "Right", "LA", "RA", "LP", "RP"] -> [w432] mode=indexing
            tunnel: w376 -> [w431] mode=indexing
            tunnel: w369 -> [w428] mode=indexing
            n257 = Number To Fractional String(number=w436) -> (F-format string=w440:string)  [unwired: 3 in]
            n258 = Number To Fractional String(number=w435) -> (F-format string=w439:string)  [unwired: 3 in]
            n259 = Number To Decimal String(number=w434) -> (decimal integer string=w438:string)  [unwired: 1 in]
            n260 = Number To Fractional String(number=w431) -> (F-format string=w430:string)  [unwired: 3 in]
            n261 = Number To Fractional String(number=w428) -> (F-format string=w429:string)  [unwired: 3 in]
            n262 = Build Array (concatenate)(w433, w432, w440, w439, w438, w430, w429) -> (w437:string[])
          }
          n263 = call <userlib>:"Open.vi"("Worksheet Name (Sheet1)"="Head Impulse", "Excel in"=w386) -> ("error out"=w395:errorcluster, "Excel out"=w396:refnum<class "Excel.lvclass">)  [unwired: 8 in]
          n264 = call <userlib>:"Write.vi"("error in (no error)"=w395, "Cell (Append to next row)"=cluster{"Row":i32, "Col":i32} {"Row"=0, "Col"=0}, "Data"=w389, "Excel in"=w396) -> ("error out"=w393:errorcluster, "Excel out"=w394:refnum<class "Excel.lvclass">)  [unwired: 5 in, 1 out]
          n265 = call <userlib>:"Write.vi"("error in (no error)"=w393, "Data"=w388, "Excel in"=w394) -> ("error out"=w392:errorcluster, "Excel out"=w391:refnum<class "Excel.lvclass">)  [unwired: 6 in, 1 out]
          n266 = call <userlib>:"Save.vi"("error in (no error)"=w392, "Excel in"=w391) -> ("Excel out"=w384:refnum<class "Excel.lvclass">)  [unwired: 7 in, 2 out]
          n267 = Bundle By Name(cluster=w385, "Excel"=w384) -> (w383:T1)
        }
        frame "Save To Excel (legacy)" {
          # "Save data to Excel in the legacy format (single row - pre 2019/08/15)"
          n268 = Unbundle By Name(w441) -> ("Excel"=w444:refnum<class "Excel.lvclass">)
          n269 = property on="Impulse Gain Method" class="Enum (strict)"() -> ("Strings []"=w463:string[], "Value"=w465:T5)  [unwired: 2 in, 2 out]
          n270 = property on="Impulse Group Gain Method" class="Enum (strict)"() -> ("Strings []"=w464:string[], "Value"=w466:T4)  [unwired: 2 in, 2 out]
          n271 = Unbundle By Name(w441) -> ("Experiment Parameters.Stimulus"=w450:string)
          n272 = Index Array(array=w463, index=w465) -> (element=w449:string)
          n273 = Index Array(array=w464, index=w466) -> (element=w448:string)
          n274 = local read "0 Gain"() -> (w467:dbl)
          n275 = local read "1 Gain"() -> (w468:dbl)
          n276 = local read "2 Gain"() -> (w469:dbl)
          n277 = local read "3 Gain"() -> (w470:dbl)
          n278 = local read "4 Gain"() -> (w471:dbl)
          n279 = local read "5 Gain"() -> (w472:dbl)
          n280 = local read "0 SD"() -> (w473:dbl)
          n281 = local read "1 SD"() -> (w474:dbl)
          n282 = local read "2 SD"() -> (w476:dbl)
          n283 = local read "3 SD"() -> (w477:dbl)
          n284 = local read "4 SD"() -> (w478:dbl)
          n285 = local read "5 SD"() -> (w475:dbl)
          n286 = Build Array(w473, w474, w476, w477, w478, w475) -> (w452:dbl[])
          n287 = Build Array(w467, w468, w469, w470, w471, w472) -> (w453:dbl[])
          n288 = local read "Patient ID"() -> (w451:string)
          n289 = Build Array (concatenate)(w453, w452) -> (w447:dbl[])
          n290 = Number To Fractional String(number=w447) -> (F-format string=w446:string[])  [unwired: 3 in]
          n291 = Build Array (concatenate)(w451, w450, w449, w448, w446) -> (w445:string[])
          n292 = call <userlib>:"Open.vi"("Worksheet Name (Sheet1)"="Head Impulse (legacy)", "Excel in"=w444) -> ("error out"=w460:errorcluster, "Excel out"=w461:refnum<class "Excel.lvclass">)  [unwired: 8 in]
          n293 = call <userlib>:"Write.vi"("error in (no error)"=w460, "Cell (Append to next row)"=cluster{"Row":i32, "Col":i32} {"Row"=0, "Col"=0}, "Data"=string[] ["Patient ID", "Stimulus", "Impulse Gain Method", "Impulse Group Method", "Left", "Right", "Left Anterior", "Right Anterior", "Left Posterior", "Right Posterior", "Left SD", "Right SD", "Left Anterior SD", "Right Anterior SD", "Left Posterior SD", "Right Posterior SD"] ("Header"), "Excel in"=w461) -> ("error out"=w456:errorcluster, "Excel out"=w457:refnum<class "Excel.lvclass">)  [unwired: 5 in, 1 out]
          n294 = call <userlib>:"Write.vi"("error in (no error)"=w456, "Data"=w445, "Excel in"=w457) -> ("error out"=w455:errorcluster, "Excel out"=w454:refnum<class "Excel.lvclass">)  [unwired: 6 in, 1 out]
          n295 = call <userlib>:"Save.vi"("error in (no error)"=w455, "Excel in"=w454) -> ("Excel out"=w443:refnum<class "Excel.lvclass">)  [unwired: 7 in, 2 out]
          n296 = Bundle By Name(cluster=w441, "Excel"=w443) -> (w442:T1)
        }
      }
    }
  }
  "Data Out" <- w1
